vi "JTAG Stim ASIC SPI Test.vi"(5 "Test Type":u16(ring) items=["SPI Self Test", "Stim Register Test", "Stim RAM Test"], 11 "error in (no error)":errorcluster) -> (6 "Test Result":string, 15 "error out":errorcluster)   [LabVIEW 2010]
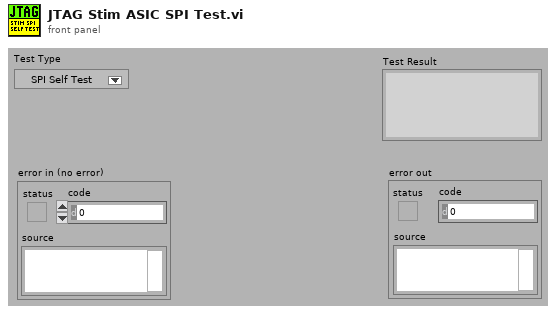
[diagram p1: front panel]
types:
  T1 = enum16{"Read General Control Registers", "Read Phase Registers", "Read RAM1", "Read RAM2", "WE Test0", "WE Test1", "WE Test2", "WE Test3", "WE Test4", "WE Test5", "WE Test6", "WE Test7", "Address Bus Test", "General Register 1's and 0's", "General Register 1's and 0's Inverse", "Phase Register 1's and 0's", "Phase Register 1's and 0's Inverse", "RAM1 data bus 0", "RAM1 data bus 1", "RAM1 data bus 2", "RAM1 data bus 3", "RAM1 data bus 4", "RAM1 data bus 5", "RAM1 data bus 6", "RAM1 data bus 7", "RAM2 data bus 0", "RAM2 data bus 1", "RAM2 data bus 2", "RAM2 data bus 3", "RAM2 data bus 4", "RAM2 data bus 5", "RAM2 data bus 6", "RAM2 data bus 7", "RAM Address Bus Test", "RAM 1's and 0's", "RAM 1's and 0's Inverse", "Address Decoder Test"}[]
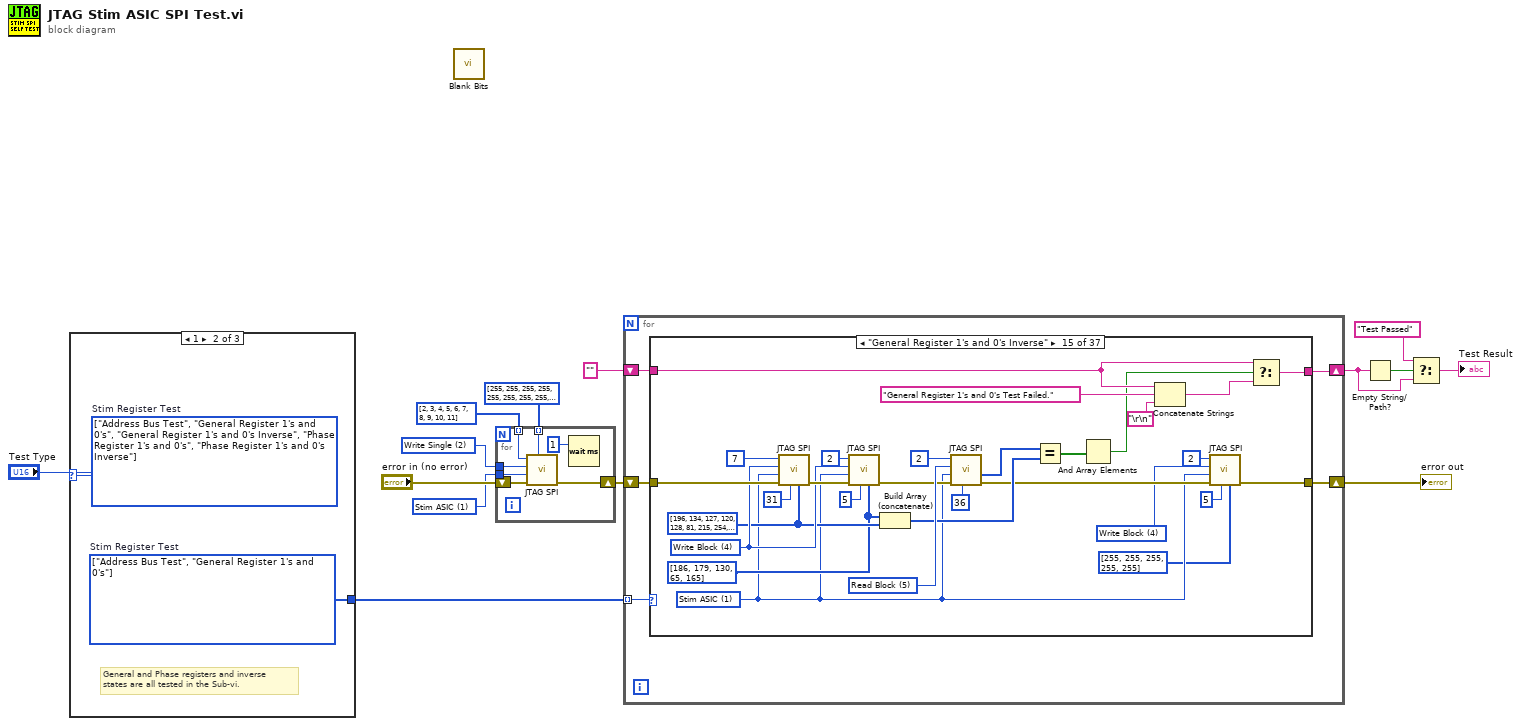
[diagram p0: block diagram]
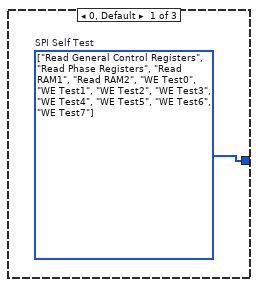
[diagram p2: hidden frame]
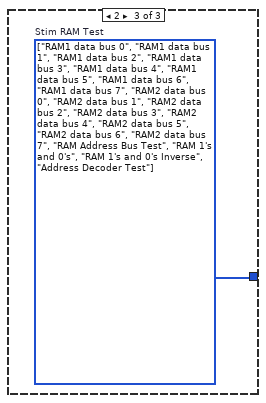
[diagram p3: hidden frame]
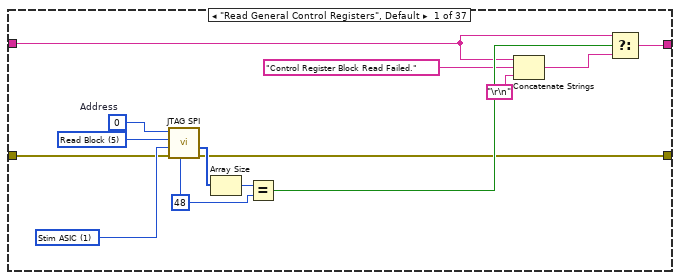
[diagram p4: hidden frame]
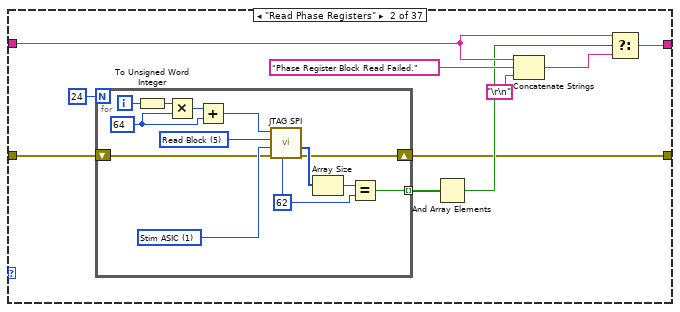
[diagram p5: hidden frame]
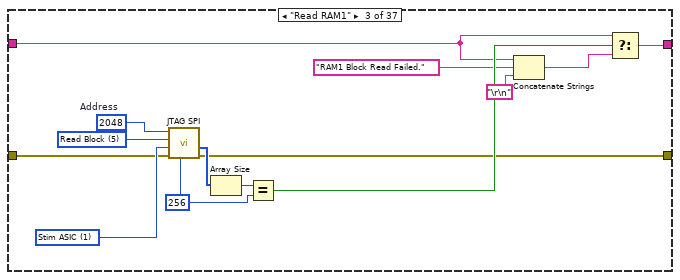
[diagram p6: hidden frame]
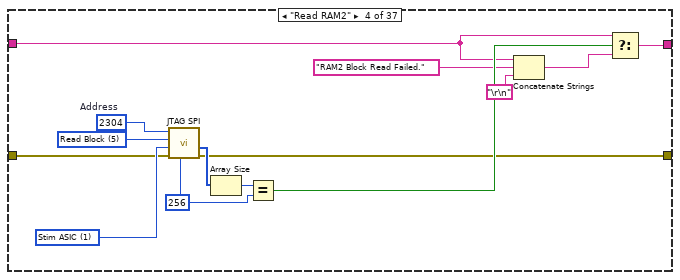
[diagram p7: hidden frame]
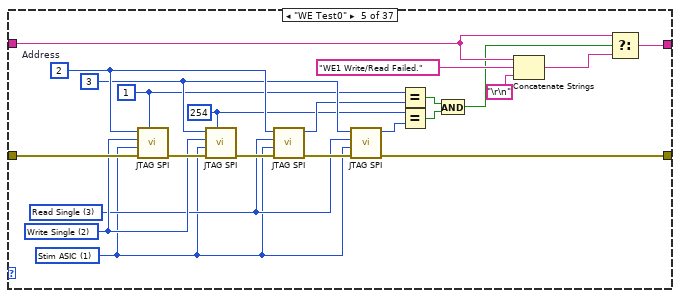
[diagram p8: hidden frame]
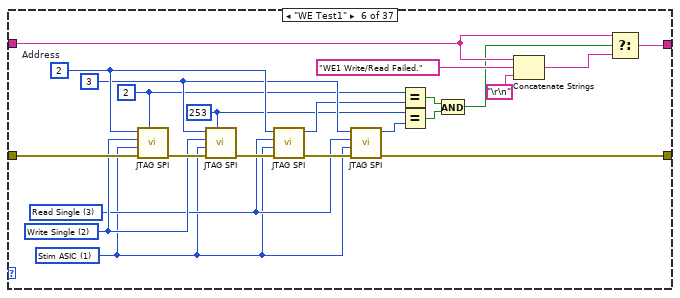
[diagram p9: hidden frame]
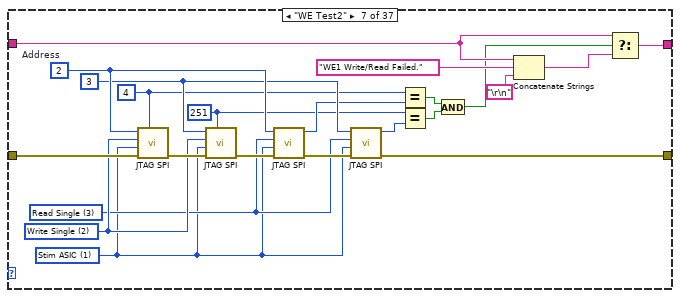
[diagram p10: hidden frame]
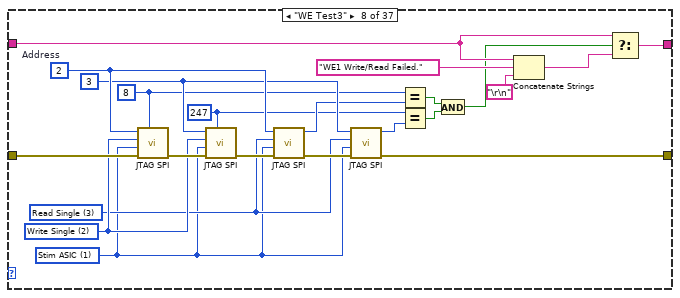
[diagram p11: hidden frame]
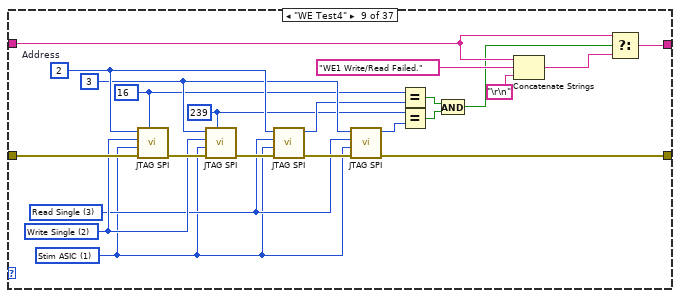
[diagram p12: hidden frame]
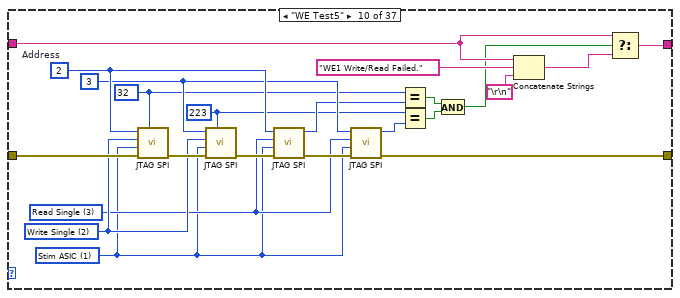
[diagram p13: hidden frame]
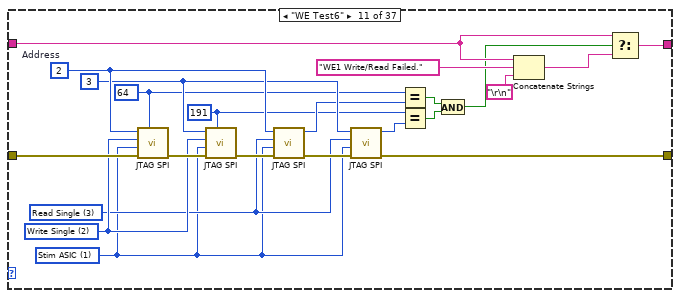
[diagram p14: hidden frame]
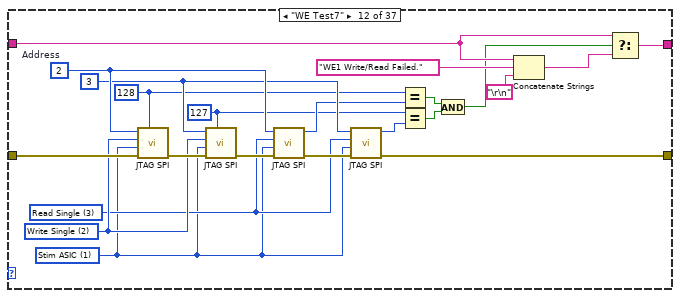
[diagram p15: hidden frame]
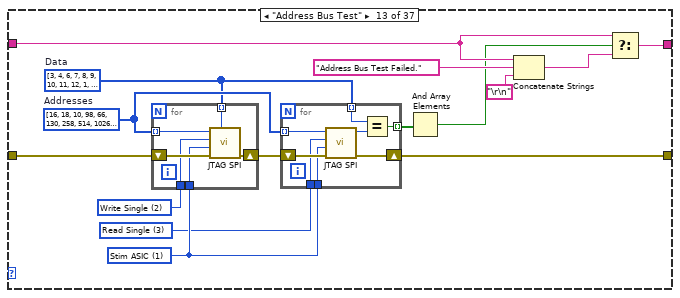
[diagram p16: hidden frame]
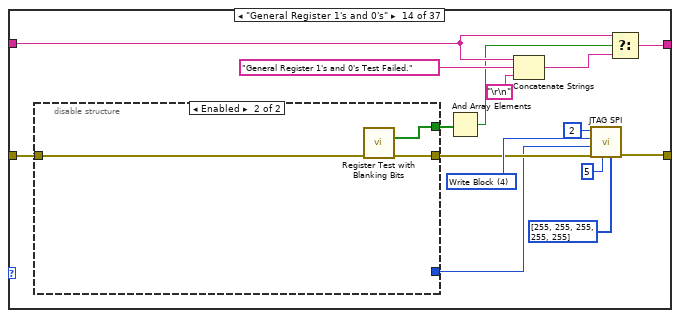
[diagram p17: hidden frame]
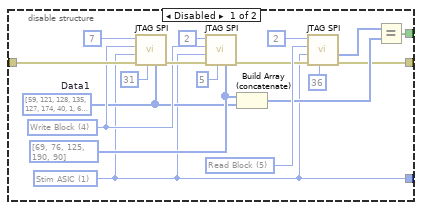
[diagram p18: hidden frame]
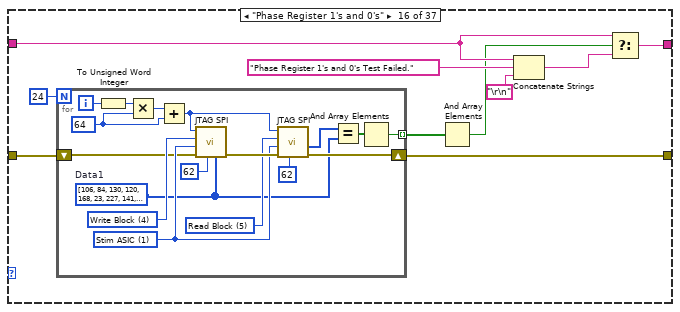
[diagram p19: hidden frame]
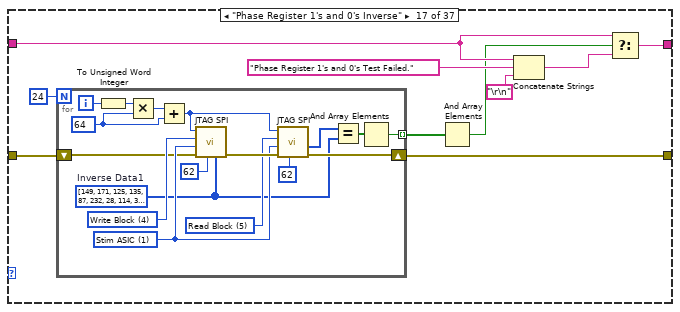
[diagram p20: hidden frame]
diagram:
  w4 = u16 2 items=["Power UP", "Power DN", "Write Single", "Read Single", "Write Block", "Read Block", "Write Masked", "Test Value"] ("Function")
  w5 = u16 1 items=["Power ASIC", "Stim ASIC", "MICS Radio", "FRAM"] ("Target")
  n1 = case shown="1" "Test Type" {
    tunnel: [w15 w16 w17] -> w7
    frame 0, Default {
      w15 = T1 [enum."Read General Control Registers", enum."Read Phase Registers", enum."Read RAM1", enum."Read RAM2", enum."WE Test0", enum."WE Test1", enum."WE Test2", enum."WE Test3", enum."WE Test4", enum."WE Test5", enum."WE Test6", enum."WE Test7"] items=["Read General Control Registers", "Read Phase Registers", "Read RAM1", "Read RAM2", "WE Test0", "WE Test1", "WE Test2", "WE Test3", "WE Test4", "WE Test5", "WE Test6", "WE Test7", "Address Bus Test", "General Register 1's and 0's", "General Register 1's and 0's Inverse", "Phase Register 1's and 0's", "Phase Register 1's and 0's Inverse", "RAM1 data bus 0", "RAM1 data bus 1", "RAM1 data bus 2", "RAM1 data bus 3", "RAM1 data bus 4", "RAM1 data bus 5", "RAM1 data bus 6", "RAM1 data bus 7", "RAM2 data bus 0", "RAM2 data bus 1", "RAM2 data bus 2", "RAM2 data bus 3", "RAM2 data bus 4", "RAM2 data bus 5", "RAM2 data bus 6", "RAM2 data bus 7", "RAM Address Bus Test", "RAM 1's and 0's", "RAM 1's and 0's Inverse", "Address Decoder Test"]  # SPI Self Test
    }
    frame 1 {
      (unwired) T1 [enum."Address Bus Test", enum."General Register 1's and 0's", enum."General Register 1's and 0's Inverse", enum."Phase Register 1's and 0's", enum."Phase Register 1's and 0's Inverse"] items=["Read General Control Registers", "Read Phase Registers", "Read RAM1", "Read RAM2", "WE Test0", "WE Test1", "WE Test2", "WE Test3", "WE Test4", "WE Test5", "WE Test6", "WE Test7", "Address Bus Test", "General Register 1's and 0's", "General Register 1's and 0's Inverse", "Phase Register 1's and 0's", "Phase Register 1's and 0's Inverse", "RAM1 data bus 0", "RAM1 data bus 1", "RAM1 data bus 2", "RAM1 data bus 3", "RAM1 data bus 4", "RAM1 data bus 5", "RAM1 data bus 6", "RAM1 data bus 7", "RAM2 data bus 0", "RAM2 data bus 1", "RAM2 data bus 2", "RAM2 data bus 3", "RAM2 data bus 4", "RAM2 data bus 5", "RAM2 data bus 6", "RAM2 data bus 7", "RAM Address Bus Test", "RAM 1's and 0's", "RAM 1's and 0's Inverse", "Address Decoder Test"]  # Stim Register Test
      w16 = T1 [enum."Address Bus Test", enum."General Register 1's and 0's"] items=["Read General Control Registers", "Read Phase Registers", "Read RAM1", "Read RAM2", "WE Test0", "WE Test1", "WE Test2", "WE Test3", "WE Test4", "WE Test5", "WE Test6", "WE Test7", "Address Bus Test", "General Register 1's and 0's", "General Register 1's and 0's Inverse", "Phase Register 1's and 0's", "Phase Register 1's and 0's Inverse", "RAM1 data bus 0", "RAM1 data bus 1", "RAM1 data bus 2", "RAM1 data bus 3", "RAM1 data bus 4", "RAM1 data bus 5", "RAM1 data bus 6", "RAM1 data bus 7", "RAM2 data bus 0", "RAM2 data bus 1", "RAM2 data bus 2", "RAM2 data bus 3", "RAM2 data bus 4", "RAM2 data bus 5", "RAM2 data bus 6", "RAM2 data bus 7", "RAM Address Bus Test", "RAM 1's and 0's", "RAM 1's and 0's Inverse", "Address Decoder Test"]  # Stim Register Test
      # "General and Phase registers and inverse\nstates are all tested in the Sub-vi."
    }
    frame 2 {
      w17 = T1 [enum."RAM1 data bus 0", enum."RAM1 data bus 1", enum."RAM1 data bus 2", enum."RAM1 data bus 3", enum."RAM1 data bus 4", enum."RAM1 data bus 5", enum."RAM1 data bus 6", enum."RAM1 data bus 7", enum."RAM2 data bus 0", enum."RAM2 data bus 1", enum."RAM2 data bus 2", enum."RAM2 data bus 3", enum."RAM2 data bus 4", enum."RAM2 data bus 5", enum."RAM2 data bus 6", enum."RAM2 data bus 7", enum."RAM Address Bus Test", enum."RAM 1's and 0's", enum."RAM 1's and 0's Inverse", enum."Address Decoder Test"] items=["Read General Control Registers", "Read Phase Registers", "Read RAM1", "Read RAM2", "WE Test0", "WE Test1", "WE Test2", "WE Test3", "WE Test4", "WE Test5", "WE Test6", "WE Test7", "Address Bus Test", "General Register 1's and 0's", "General Register 1's and 0's Inverse", "Phase Register 1's and 0's", "Phase Register 1's and 0's Inverse", "RAM1 data bus 0", "RAM1 data bus 1", "RAM1 data bus 2", "RAM1 data bus 3", "RAM1 data bus 4", "RAM1 data bus 5", "RAM1 data bus 6", "RAM1 data bus 7", "RAM2 data bus 0", "RAM2 data bus 1", "RAM2 data bus 2", "RAM2 data bus 3", "RAM2 data bus 4", "RAM2 data bus 5", "RAM2 data bus 6", "RAM2 data bus 7", "RAM Address Bus Test", "RAM 1's and 0's", "RAM 1's and 0's Inverse", "Address Decoder Test"]  # Stim RAM Test
    }
  }
  n2 = call "Blank Bits.vi"() -> ()  [unwired: 14 in, 2 out]
  n3 = for {
    tunnel: w5 -> [w22]
    tunnel: w4 -> [w21]
    shift-right: [w23] -> w1
    shift-left: "error in (no error)" -> [w24]
    tunnel: u8[] [255, 255, 255, 255, 255, 255, 255, 255, 63, 3] ("Block Write Data") -> [w20] mode=indexing
    tunnel: u16[] [2, 3, 4, 5, 6, 7, 8, 9, 10, 11] ("Block Write Data") -> [w19] mode=indexing
    n4 = call "JTAG SPI.vi"("Value"=w20, "error in (no error)"=w24, "Target"=w22, "Function"=w21, "Address"=w19) -> ("error out"=w23:errorcluster)  [unwired: 3 in, 3 out]
    n5 = Wait (ms)(milliseconds to wait=u32 1) -> ()  [unwired: 1 out]
  }
  n6 = for {
    tunnel: w7 -> [w29] mode=indexing
    shift-right: [w27] -> w11
    shift-left: "" -> [w26]
    shift-right: [w25] -> w13
    shift-left: w1 -> [w28]
    n7 = case shown="\"General Register 1's and 0's Inverse\"" w29 {
      tunnel: w28 -> [w37 w53 w74 w88 w116 w138 w160 w182 w204 w226 w248 w270 w285 w314 w364 w367 w394 w440 w462 w484 w506 w528 w550 w572 w594 w616 w638 w660 w682 w704 w726 w748 w770 w785 w813 w831 w865]
      tunnel: [w30 w44 w67 w81 w106 w128 w150 w172 w194 w216 w238 w260 w275 w301 w339 w366 w393 w430 w452 w474 w496 w518 w540 w562 w584 w606 w628 w650 w672 w694 w716 w738 w760 w775 w812 w830 w852] -> w25
      tunnel: [w36 w52 w73 w87 w115 w137 w159 w181 w203 w225 w247 w269 w284 w313 w363 w374 w401 w439 w461 w483 w505 w527 w549 w571 w593 w615 w637 w659 w681 w703 w725 w747 w769 w784 w819 w837 w864] -> w27
      tunnel: w26 -> [w34 w50 w71 w85 w113 w135 w157 w179 w201 w223 w245 w267 w283 w312 w362 w373 w400 w437 w459 w481 w503 w525 w547 w569 w591 w613 w635 w657 w679 w701 w723 w745 w767 w783 w818 w836 w863]
      frame "Read General Control Registers", Default {
        w38 = u16 48 ("Blocksize")
        w41 = u16 1 items=["Power ASIC", "Stim ASIC", "MICS Radio", "FRAM"] ("Target")
        w42 = u16 5 items=["Power UP", "Power DN", "Write Single", "Read Single", "Write Block", "Read Block", "Write Masked", "Test Value"] ("Function")
        w43 = u16 0  # Address
        n8 = call "JTAG SPI.vi"("Blocksize"=w38, "error in (no error)"=w37, "Target"=w41, "Function"=w42, "Address"=w43) -> ("error out"=w30:errorcluster, "Block Read Data"=w40:u16[])  [unwired: 3 in, 2 out]
        n9 = Array Size(array=w40) -> (size(s)=w39:i32)
        n10 = Equal?(x=w39, y=w38) -> (x = y?=w35:bool)
        n11 = Concatenate Strings(w34, "Control Register Block Read Failed." ("string"), "\r\n") -> (w33:string)
        n12 = Select(t=w34, s=w35, f=w33) -> (s? t:f=w36:string)
      }
      frame "Read Phase Registers" {
        n13 = for {
          N: 24 -> [_]
          tunnel: [w59] -> w51 mode=indexing
          shift-right: [w60] -> w44
          shift-left: w53 -> [w61]
          i -> [w58]
          w55 = u16 64 ("y")
          w62 = u16 62 ("Blocksize")
          w65 = u16 1 items=["Power ASIC", "Stim ASIC", "MICS Radio", "FRAM"] ("Target")
          w66 = u16 5 items=["Power UP", "Power DN", "Write Single", "Read Single", "Write Block", "Read Block", "Write Masked", "Test Value"] ("Function")
          n14 = To Unsigned Word Integer(number=w58) -> (unsigned 16bit integer=w57:u16)
          n15 = Multiply(x=w57, y=w55) -> (x*y=w56:u16)
          n16 = Add(x=w56, y=w55) -> (x+y=w54:u16)
          n17 = call "JTAG SPI.vi"("Blocksize"=w62, "error in (no error)"=w61, "Target"=w65, "Function"=w66, "Address"=w54) -> ("error out"=w60:errorcluster, "Block Read Data"=w64:u16[])  [unwired: 3 in, 2 out]
          n18 = Array Size(array=w64) -> (size(s)=w63:i32)
          n19 = Equal?(x=w63, y=w62) -> (x = y?=w59:bool)
        }
        n20 = And Array Elements(Boolean array=w51) -> (logical AND=w46:bool)
        n21 = Concatenate Strings(w50, "Phase Register Block Read Failed." ("string"), "\r\n") -> (w49:string)
        n22 = Select(t=w50, s=w46, f=w49) -> (s? t:f=w52:string)
      }
      frame "Read RAM1" {
        w75 = u16 256 ("Blocksize")
        w78 = u16 1 items=["Power ASIC", "Stim ASIC", "MICS Radio", "FRAM"] ("Target")
        w79 = u16 5 items=["Power UP", "Power DN", "Write Single", "Read Single", "Write Block", "Read Block", "Write Masked", "Test Value"] ("Function")
        w80 = u16 2048  # Address
        n23 = call "JTAG SPI.vi"("Blocksize"=w75, "error in (no error)"=w74, "Target"=w78, "Function"=w79, "Address"=w80) -> ("error out"=w67:errorcluster, "Block Read Data"=w77:u16[])  [unwired: 3 in, 2 out]
        n24 = Array Size(array=w77) -> (size(s)=w76:i32)
        n25 = Equal?(x=w76, y=w75) -> (x = y?=w72:bool)
        n26 = Concatenate Strings(w71, "RAM1 Block Read Failed." ("string"), "\r\n") -> (w70:string)
        n27 = Select(t=w71, s=w72, f=w70) -> (s? t:f=w73:string)
      }
      frame "Read RAM2" {
        w89 = u16 256 ("Blocksize")
        w92 = u16 1 items=["Power ASIC", "Stim ASIC", "MICS Radio", "FRAM"] ("Target")
        w93 = u16 5 items=["Power UP", "Power DN", "Write Single", "Read Single", "Write Block", "Read Block", "Write Masked", "Test Value"] ("Function")
        w94 = u16 2304  # Address
        n28 = call "JTAG SPI.vi"("Blocksize"=w89, "error in (no error)"=w88, "Target"=w92, "Function"=w93, "Address"=w94) -> ("error out"=w81:errorcluster, "Block Read Data"=w91:u16[])  [unwired: 3 in, 2 out]
        n29 = Array Size(array=w91) -> (size(s)=w90:i32)
        n30 = Equal?(x=w90, y=w89) -> (x = y?=w86:bool)
        n31 = Concatenate Strings(w85, "RAM2 Block Read Failed." ("string"), "\r\n") -> (w84:string)
        n32 = Select(t=w85, s=w86, f=w84) -> (s? t:f=w87:string)
      }
      frame "WE Test0" {
        w98 = u8 254 ("Value")
        w100 = u8 1 ("Value")
        w102 = u16 3 items=["Power UP", "Power DN", "Write Single", "Read Single", "Write Block", "Read Block", "Write Masked", "Test Value"] ("Function")
        w104 = u16 3 ("Address")
        w101 = u16 1 items=["Power ASIC", "Stim ASIC", "MICS Radio", "FRAM"] ("Target")
        w103 = u16 2 items=["Power UP", "Power DN", "Write Single", "Read Single", "Write Block", "Read Block", "Write Masked", "Test Value"] ("Function")
        w105 = u16 2  # Address
        n33 = call "JTAG SPI.vi"("Value"=w100, "error in (no error)"=w116, "Target"=w101, "Function"=w103, "Address"=w105) -> ("error out"=w109:errorcluster)  [unwired: 3 in, 3 out]
        n34 = call "JTAG SPI.vi"("Value"=w98, "error in (no error)"=w109, "Target"=w101, "Function"=w103, "Address"=w104) -> ("error out"=w108:errorcluster)  [unwired: 3 in, 3 out]
        n35 = call "JTAG SPI.vi"("error in (no error)"=w108, "Target"=w101, "Function"=w102, "Address"=w105) -> ("error out"=w107:errorcluster, "Read Value"=w99:u8)  [unwired: 4 in, 2 out]
        n36 = call "JTAG SPI.vi"("error in (no error)"=w107, "Target"=w101, "Function"=w102, "Address"=w104) -> ("error out"=w106:errorcluster, "Read Value"=w97:u8)  [unwired: 4 in, 2 out]
        n37 = Equal?(x=w100, y=w99) -> (x = y?=w95:bool)
        n38 = Equal?(x=w98, y=w97) -> (x = y?=w114:bool)
        n39 = And(x=w95, y=w114) -> (x .and. y?=w96:bool)
        n40 = Concatenate Strings(w113, "WE1 Write/Read Failed." ("string"), "\r\n") -> (w112:string)
        n41 = Select(t=w113, s=w96, f=w112) -> (s? t:f=w115:string)
      }
      frame "WE Test1" {
        w120 = u8 253 ("Value")
        w122 = u8 2 ("Value")
        w124 = u16 3 items=["Power UP", "Power DN", "Write Single", "Read Single", "Write Block", "Read Block", "Write Masked", "Test Value"] ("Function")
        w126 = u16 3 ("Address")
        w123 = u16 1 items=["Power ASIC", "Stim ASIC", "MICS Radio", "FRAM"] ("Target")
        w125 = u16 2 items=["Power UP", "Power DN", "Write Single", "Read Single", "Write Block", "Read Block", "Write Masked", "Test Value"] ("Function")
        w127 = u16 2  # Address
        n42 = call "JTAG SPI.vi"("Value"=w122, "error in (no error)"=w138, "Target"=w123, "Function"=w125, "Address"=w127) -> ("error out"=w131:errorcluster)  [unwired: 3 in, 3 out]
        n43 = call "JTAG SPI.vi"("Value"=w120, "error in (no error)"=w131, "Target"=w123, "Function"=w125, "Address"=w126) -> ("error out"=w130:errorcluster)  [unwired: 3 in, 3 out]
        n44 = call "JTAG SPI.vi"("error in (no error)"=w130, "Target"=w123, "Function"=w124, "Address"=w127) -> ("error out"=w129:errorcluster, "Read Value"=w121:u8)  [unwired: 4 in, 2 out]
        n45 = call "JTAG SPI.vi"("error in (no error)"=w129, "Target"=w123, "Function"=w124, "Address"=w126) -> ("error out"=w128:errorcluster, "Read Value"=w119:u8)  [unwired: 4 in, 2 out]
        n46 = Equal?(x=w122, y=w121) -> (x = y?=w117:bool)
        n47 = Equal?(x=w120, y=w119) -> (x = y?=w136:bool)
        n48 = And(x=w117, y=w136) -> (x .and. y?=w118:bool)
        n49 = Concatenate Strings(w135, "WE1 Write/Read Failed." ("string"), "\r\n") -> (w134:string)
        n50 = Select(t=w135, s=w118, f=w134) -> (s? t:f=w137:string)
      }
      frame "WE Test2" {
        w142 = u8 251 ("Value")
        w144 = u8 4 ("Value")
        w146 = u16 3 items=["Power UP", "Power DN", "Write Single", "Read Single", "Write Block", "Read Block", "Write Masked", "Test Value"] ("Function")
        w148 = u16 3 ("Address")
        w145 = u16 1 items=["Power ASIC", "Stim ASIC", "MICS Radio", "FRAM"] ("Target")
        w147 = u16 2 items=["Power UP", "Power DN", "Write Single", "Read Single", "Write Block", "Read Block", "Write Masked", "Test Value"] ("Function")
        w149 = u16 2  # Address
        n51 = call "JTAG SPI.vi"("Value"=w144, "error in (no error)"=w160, "Target"=w145, "Function"=w147, "Address"=w149) -> ("error out"=w153:errorcluster)  [unwired: 3 in, 3 out]
        n52 = call "JTAG SPI.vi"("Value"=w142, "error in (no error)"=w153, "Target"=w145, "Function"=w147, "Address"=w148) -> ("error out"=w152:errorcluster)  [unwired: 3 in, 3 out]
        n53 = call "JTAG SPI.vi"("error in (no error)"=w152, "Target"=w145, "Function"=w146, "Address"=w149) -> ("error out"=w151:errorcluster, "Read Value"=w143:u8)  [unwired: 4 in, 2 out]
        n54 = call "JTAG SPI.vi"("error in (no error)"=w151, "Target"=w145, "Function"=w146, "Address"=w148) -> ("error out"=w150:errorcluster, "Read Value"=w141:u8)  [unwired: 4 in, 2 out]
        n55 = Equal?(x=w144, y=w143) -> (x = y?=w139:bool)
        n56 = Equal?(x=w142, y=w141) -> (x = y?=w158:bool)
        n57 = And(x=w139, y=w158) -> (x .and. y?=w140:bool)
        n58 = Concatenate Strings(w157, "WE1 Write/Read Failed." ("string"), "\r\n") -> (w156:string)
        n59 = Select(t=w157, s=w140, f=w156) -> (s? t:f=w159:string)
      }
      frame "WE Test3" {
        w164 = u8 247 ("Value")
        w166 = u8 8 ("Value")
        w168 = u16 3 items=["Power UP", "Power DN", "Write Single", "Read Single", "Write Block", "Read Block", "Write Masked", "Test Value"] ("Function")
        w170 = u16 3 ("Address")
        w167 = u16 1 items=["Power ASIC", "Stim ASIC", "MICS Radio", "FRAM"] ("Target")
        w169 = u16 2 items=["Power UP", "Power DN", "Write Single", "Read Single", "Write Block", "Read Block", "Write Masked", "Test Value"] ("Function")
        w171 = u16 2  # Address
        n60 = call "JTAG SPI.vi"("Value"=w166, "error in (no error)"=w182, "Target"=w167, "Function"=w169, "Address"=w171) -> ("error out"=w175:errorcluster)  [unwired: 3 in, 3 out]
        n61 = call "JTAG SPI.vi"("Value"=w164, "error in (no error)"=w175, "Target"=w167, "Function"=w169, "Address"=w170) -> ("error out"=w174:errorcluster)  [unwired: 3 in, 3 out]
        n62 = call "JTAG SPI.vi"("error in (no error)"=w174, "Target"=w167, "Function"=w168, "Address"=w171) -> ("error out"=w173:errorcluster, "Read Value"=w165:u8)  [unwired: 4 in, 2 out]
        n63 = call "JTAG SPI.vi"("error in (no error)"=w173, "Target"=w167, "Function"=w168, "Address"=w170) -> ("error out"=w172:errorcluster, "Read Value"=w163:u8)  [unwired: 4 in, 2 out]
        n64 = Equal?(x=w166, y=w165) -> (x = y?=w161:bool)
        n65 = Equal?(x=w164, y=w163) -> (x = y?=w180:bool)
        n66 = And(x=w161, y=w180) -> (x .and. y?=w162:bool)
        n67 = Concatenate Strings(w179, "WE1 Write/Read Failed." ("string"), "\r\n") -> (w178:string)
        n68 = Select(t=w179, s=w162, f=w178) -> (s? t:f=w181:string)
      }
      frame "WE Test4" {
        w186 = u8 239 ("Value")
        w188 = u8 16 ("Value")
        w190 = u16 3 items=["Power UP", "Power DN", "Write Single", "Read Single", "Write Block", "Read Block", "Write Masked", "Test Value"] ("Function")
        w192 = u16 3 ("Address")
        w189 = u16 1 items=["Power ASIC", "Stim ASIC", "MICS Radio", "FRAM"] ("Target")
        w191 = u16 2 items=["Power UP", "Power DN", "Write Single", "Read Single", "Write Block", "Read Block", "Write Masked", "Test Value"] ("Function")
        w193 = u16 2  # Address
        n69 = call "JTAG SPI.vi"("Value"=w188, "error in (no error)"=w204, "Target"=w189, "Function"=w191, "Address"=w193) -> ("error out"=w197:errorcluster)  [unwired: 3 in, 3 out]
        n70 = call "JTAG SPI.vi"("Value"=w186, "error in (no error)"=w197, "Target"=w189, "Function"=w191, "Address"=w192) -> ("error out"=w196:errorcluster)  [unwired: 3 in, 3 out]
        n71 = call "JTAG SPI.vi"("error in (no error)"=w196, "Target"=w189, "Function"=w190, "Address"=w193) -> ("error out"=w195:errorcluster, "Read Value"=w187:u8)  [unwired: 4 in, 2 out]
        n72 = call "JTAG SPI.vi"("error in (no error)"=w195, "Target"=w189, "Function"=w190, "Address"=w192) -> ("error out"=w194:errorcluster, "Read Value"=w185:u8)  [unwired: 4 in, 2 out]
        n73 = Equal?(x=w188, y=w187) -> (x = y?=w183:bool)
        n74 = Equal?(x=w186, y=w185) -> (x = y?=w202:bool)
        n75 = And(x=w183, y=w202) -> (x .and. y?=w184:bool)
        n76 = Concatenate Strings(w201, "WE1 Write/Read Failed." ("string"), "\r\n") -> (w200:string)
        n77 = Select(t=w201, s=w184, f=w200) -> (s? t:f=w203:string)
      }
      frame "WE Test5" {
        w208 = u8 223 ("Value")
        w210 = u8 32 ("Value")
        w212 = u16 3 items=["Power UP", "Power DN", "Write Single", "Read Single", "Write Block", "Read Block", "Write Masked", "Test Value"] ("Function")
        w214 = u16 3 ("Address")
        w211 = u16 1 items=["Power ASIC", "Stim ASIC", "MICS Radio", "FRAM"] ("Target")
        w213 = u16 2 items=["Power UP", "Power DN", "Write Single", "Read Single", "Write Block", "Read Block", "Write Masked", "Test Value"] ("Function")
        w215 = u16 2  # Address
        n78 = call "JTAG SPI.vi"("Value"=w210, "error in (no error)"=w226, "Target"=w211, "Function"=w213, "Address"=w215) -> ("error out"=w219:errorcluster)  [unwired: 3 in, 3 out]
        n79 = call "JTAG SPI.vi"("Value"=w208, "error in (no error)"=w219, "Target"=w211, "Function"=w213, "Address"=w214) -> ("error out"=w218:errorcluster)  [unwired: 3 in, 3 out]
        n80 = call "JTAG SPI.vi"("error in (no error)"=w218, "Target"=w211, "Function"=w212, "Address"=w215) -> ("error out"=w217:errorcluster, "Read Value"=w209:u8)  [unwired: 4 in, 2 out]
        n81 = call "JTAG SPI.vi"("error in (no error)"=w217, "Target"=w211, "Function"=w212, "Address"=w214) -> ("error out"=w216:errorcluster, "Read Value"=w207:u8)  [unwired: 4 in, 2 out]
        n82 = Equal?(x=w210, y=w209) -> (x = y?=w205:bool)
        n83 = Equal?(x=w208, y=w207) -> (x = y?=w224:bool)
        n84 = And(x=w205, y=w224) -> (x .and. y?=w206:bool)
        n85 = Concatenate Strings(w223, "WE1 Write/Read Failed." ("string"), "\r\n") -> (w222:string)
        n86 = Select(t=w223, s=w206, f=w222) -> (s? t:f=w225:string)
      }
      frame "WE Test6" {
        w230 = u8 191 ("Value")
        w232 = u8 64 ("Value")
        w234 = u16 3 items=["Power UP", "Power DN", "Write Single", "Read Single", "Write Block", "Read Block", "Write Masked", "Test Value"] ("Function")
        w236 = u16 3 ("Address")
        w233 = u16 1 items=["Power ASIC", "Stim ASIC", "MICS Radio", "FRAM"] ("Target")
        w235 = u16 2 items=["Power UP", "Power DN", "Write Single", "Read Single", "Write Block", "Read Block", "Write Masked", "Test Value"] ("Function")
        w237 = u16 2  # Address
        n87 = call "JTAG SPI.vi"("Value"=w232, "error in (no error)"=w248, "Target"=w233, "Function"=w235, "Address"=w237) -> ("error out"=w241:errorcluster)  [unwired: 3 in, 3 out]
        n88 = call "JTAG SPI.vi"("Value"=w230, "error in (no error)"=w241, "Target"=w233, "Function"=w235, "Address"=w236) -> ("error out"=w240:errorcluster)  [unwired: 3 in, 3 out]
        n89 = call "JTAG SPI.vi"("error in (no error)"=w240, "Target"=w233, "Function"=w234, "Address"=w237) -> ("error out"=w239:errorcluster, "Read Value"=w231:u8)  [unwired: 4 in, 2 out]
        n90 = call "JTAG SPI.vi"("error in (no error)"=w239, "Target"=w233, "Function"=w234, "Address"=w236) -> ("error out"=w238:errorcluster, "Read Value"=w229:u8)  [unwired: 4 in, 2 out]
        n91 = Equal?(x=w232, y=w231) -> (x = y?=w227:bool)
        n92 = Equal?(x=w230, y=w229) -> (x = y?=w246:bool)
        n93 = And(x=w227, y=w246) -> (x .and. y?=w228:bool)
        n94 = Concatenate Strings(w245, "WE1 Write/Read Failed." ("string"), "\r\n") -> (w244:string)
        n95 = Select(t=w245, s=w228, f=w244) -> (s? t:f=w247:string)
      }
      frame "WE Test7" {
        w252 = u8 127 ("Value")
        w254 = u8 128 ("Value")
        w256 = u16 3 items=["Power UP", "Power DN", "Write Single", "Read Single", "Write Block", "Read Block", "Write Masked", "Test Value"] ("Function")
        w258 = u16 3 ("Address")
        w255 = u16 1 items=["Power ASIC", "Stim ASIC", "MICS Radio", "FRAM"] ("Target")
        w257 = u16 2 items=["Power UP", "Power DN", "Write Single", "Read Single", "Write Block", "Read Block", "Write Masked", "Test Value"] ("Function")
        w259 = u16 2  # Address
        n96 = call "JTAG SPI.vi"("Value"=w254, "error in (no error)"=w270, "Target"=w255, "Function"=w257, "Address"=w259) -> ("error out"=w263:errorcluster)  [unwired: 3 in, 3 out]
        n97 = call "JTAG SPI.vi"("Value"=w252, "error in (no error)"=w263, "Target"=w255, "Function"=w257, "Address"=w258) -> ("error out"=w262:errorcluster)  [unwired: 3 in, 3 out]
        n98 = call "JTAG SPI.vi"("error in (no error)"=w262, "Target"=w255, "Function"=w256, "Address"=w259) -> ("error out"=w261:errorcluster, "Read Value"=w253:u8)  [unwired: 4 in, 2 out]
        n99 = call "JTAG SPI.vi"("error in (no error)"=w261, "Target"=w255, "Function"=w256, "Address"=w258) -> ("error out"=w260:errorcluster, "Read Value"=w251:u8)  [unwired: 4 in, 2 out]
        n100 = Equal?(x=w254, y=w253) -> (x = y?=w249:bool)
        n101 = Equal?(x=w252, y=w251) -> (x = y?=w268:bool)
        n102 = And(x=w249, y=w268) -> (x .and. y?=w250:bool)
        n103 = Concatenate Strings(w267, "WE1 Write/Read Failed." ("string"), "\r\n") -> (w266:string)
        n104 = Select(t=w267, s=w250, f=w266) -> (s? t:f=w269:string)
      }
      frame "Address Bus Test" {
        w274 = u16[] [16, 18, 10, 98, 66, 130, 258, 514, 1026, 2, 3, 6]  # Addresses
        w273 = u8[] [3, 4, 6, 7, 8, 9, 10, 11, 12, 1, 2, 5]  # Data
        w276 = u16 3 items=["Power UP", "Power DN", "Write Single", "Read Single", "Write Block", "Read Block", "Write Masked", "Test Value"] ("Function")
        w277 = u16 1 items=["Power ASIC", "Stim ASIC", "MICS Radio", "FRAM"] ("Target")
        w278 = u16 2 items=["Power UP", "Power DN", "Write Single", "Read Single", "Write Block", "Read Block", "Write Masked", "Test Value"] ("Function")
        n105 = for {
          tunnel: w274 -> [w297] mode=indexing
          tunnel: w278 -> [w296]
          tunnel: w277 -> [w295]
          tunnel: w273 -> [w294] mode=indexing
          shift-right: [w298] -> w279
          shift-left: w285 -> [w299]
          n106 = call "JTAG SPI.vi"("Value"=w294, "error in (no error)"=w299, "Target"=w295, "Function"=w296, "Address"=w297) -> ("error out"=w298:errorcluster)  [unwired: 3 in, 3 out]
        }
        n107 = for {
          tunnel: w277 -> [w292]
          tunnel: w276 -> [w291]
          shift-right: [w290] -> w275
          shift-left: w279 -> [w293]
          tunnel: w274 -> [w289] mode=indexing
          tunnel: w273 -> [w287] mode=indexing
          tunnel: [w286] -> w272 mode=indexing
          n108 = call "JTAG SPI.vi"("error in (no error)"=w293, "Target"=w292, "Function"=w291, "Address"=w289) -> ("error out"=w290:errorcluster, "Read Value"=w288:u8)  [unwired: 4 in, 2 out]
          n109 = Equal?(x=w287, y=w288) -> (x = y?=w286:bool)
        }
        n110 = And Array Elements(Boolean array=w272) -> (logical AND=w271:bool)
        n111 = Concatenate Strings(w283, "Address Bus Test Failed." ("string"), "\r\n") -> (w282:string)
        n112 = Select(t=w283, s=w271, f=w282) -> (s? t:f=w284:string)
      }
      frame "General Register 1's and 0's" {
        w304 = u16 4 items=["Power UP", "Power DN", "Write Single", "Read Single", "Write Block", "Read Block", "Write Masked", "Test Value"] ("Function")
        n113 = disable-structure shown="Enabled" {
          disable-tunnel: w314 -> [w332 w335]
          disable-tunnel: [w330 w333] -> w308
          disable-tunnel: [w316 w334] -> w302
          disable-tunnel: [w315 _] -> w300
          frame Disabled {
            w320 = u8[] [69, 76, 125, 190, 90] ("Data")
            w319 = u8[] [59, 121, 128, 135, 127, 174, 40, 1, 69, 137, 97, 116, 28, 20, 222, 248, 188, 218, 225, 189, 56, 57, 170, 225, 160, 126, 169, 73, 216, 60, 26]  # Data1
            w331 = u16 5 items=["Power UP", "Power DN", "Write Single", "Read Single", "Write Block", "Read Block", "Write Masked", "Test Value"] ("Function")
            w315 = u16 1 items=["Power ASIC", "Stim ASIC", "MICS Radio", "FRAM"] ("Target")
            w325 = u16 4 items=["Power UP", "Power DN", "Write Single", "Read Single", "Write Block", "Read Block", "Write Masked", "Test Value"] ("Function")
            n114 = call "JTAG SPI.vi"("Block Write Data"=w319, "Blocksize"=u16 31, "error in (no error)"=w332, "Target"=w315, "Function"=w325, "Address"=u16 7) -> ("error out"=w327:errorcluster)  [unwired: 2 in, 3 out]
            n115 = call "JTAG SPI.vi"("Block Write Data"=w320, "Blocksize"=u16 5, "error in (no error)"=w327, "Target"=w315, "Function"=w325, "Address"=u16 2) -> ("error out"=w322:errorcluster)  [unwired: 2 in, 3 out]
            n116 = Build Array (concatenate)(w320, w319) -> (w317:u8[])
            n117 = call "JTAG SPI.vi"("Blocksize"=u16 36, "error in (no error)"=w322, "Target"=w315, "Function"=w331, "Address"=u16 2) -> ("error out"=w316:errorcluster, "Block Read Data"=w318:u16[])  [unwired: 3 in, 2 out]
            n118 = Equal?(x=w318, y=w317) -> (x = y?=w330:bool[])
          }
          frame Enabled {
            n119 = call "Register Test with Blanking Bits.vi"("error in"=w335) -> ("Readback Match?"=w333:bool[], "error out"=w334:errorcluster)  [unwired: 13 in]
          }
        }
        n120 = And Array Elements(Boolean array=w308) -> (logical AND=w307:bool)
        n121 = Concatenate Strings(w312, "General Register 1's and 0's Test Failed." ("string"), "\r\n") -> (w311:string)
        n122 = call "JTAG SPI.vi"("Block Write Data"=u8[] [255, 255, 255, 255, 255] ("Inverse Data2"), "Blocksize"=u16 5, "error in (no error)"=w302, "Target"=w300, "Function"=w304, "Address"=u16 2) -> ("error out"=w301:errorcluster)  [unwired: 2 in, 3 out]
        n123 = Select(t=w312, s=w307, f=w311) -> (s? t:f=w313:string)
      }
      frame "General Register 1's and 0's Inverse" {
        w338 = u16 4 items=["Power UP", "Power DN", "Write Single", "Read Single", "Write Block", "Read Block", "Write Masked", "Test Value"] ("Function")
        w343 = u8[] [186, 179, 130, 65, 165] ("Inverse Data2")
        w344 = u8[] [196, 134, 127, 120, 128, 81, 215, 254, 186, 118, 158, 139, 227, 235, 33, 7, 67, 37, 30, 66, 199, 198, 85, 30, 95, 129, 86, 182, 39, 195, 229] ("Inverse Data1")
        w358 = u16 5 items=["Power UP", "Power DN", "Write Single", "Read Single", "Write Block", "Read Block", "Write Masked", "Test Value"] ("Function")
        w337 = u16 1 items=["Power ASIC", "Stim ASIC", "MICS Radio", "FRAM"] ("Target")
        w351 = u16 4 items=["Power UP", "Power DN", "Write Single", "Read Single", "Write Block", "Read Block", "Write Masked", "Test Value"] ("Function")
        n124 = call "JTAG SPI.vi"("Block Write Data"=w344, "Blocksize"=u16 31, "error in (no error)"=w364, "Target"=w337, "Function"=w351, "Address"=u16 7) -> ("error out"=w353:errorcluster)  [unwired: 2 in, 3 out]
        n125 = call "JTAG SPI.vi"("Block Write Data"=w343, "Blocksize"=u16 5, "error in (no error)"=w353, "Target"=w337, "Function"=w351, "Address"=u16 2) -> ("error out"=w348:errorcluster)  [unwired: 2 in, 3 out]
        n126 = Build Array (concatenate)(w343, w344) -> (w345:u8[])
        n127 = call "JTAG SPI.vi"("Blocksize"=u16 36, "error in (no error)"=w348, "Target"=w337, "Function"=w358, "Address"=u16 2) -> ("error out"=w340:errorcluster, "Block Read Data"=w346:u16[])  [unwired: 3 in, 2 out]
        n128 = Equal?(x=w346, y=w345) -> (x = y?=w357:bool[])
        n129 = And Array Elements(Boolean array=w357) -> (logical AND=w356:bool)
        n130 = Concatenate Strings(w362, "General Register 1's and 0's Test Failed." ("string"), "\r\n") -> (w361:string)
        n131 = call "JTAG SPI.vi"("Block Write Data"=u8[] [255, 255, 255, 255, 255] ("Inverse Data2"), "Blocksize"=u16 5, "error in (no error)"=w340, "Target"=w337, "Function"=w338, "Address"=u16 2) -> ("error out"=w339:errorcluster)  [unwired: 2 in, 3 out]
        n132 = Select(t=w362, s=w356, f=w361) -> (s? t:f=w363:string)
      }
      frame "Phase Register 1's and 0's" {
        n133 = for {
          N: 24 -> [_]
          shift-right: [w379] -> w366
          shift-left: w367 -> [w380]
          tunnel: [w375] -> w365 mode=indexing
          i -> [w391]
          w377 = u8[] [106, 84, 130, 120, 168, 23, 227, 141, 252, 8, 179, 118, 214, 187, 218, 212, 173, 207, 30, 186, 226, 198, 106, 248, 43, 21, 191, 233, 243, 156, 193, 243, 252, 127, 153, 110, 12, 64, 120, 1, 41, 97, 179, 189, 235, 149, 31, 156, 10, 101, 84, 144, 102, 8, 15, 123, 212, 23, 29, 5, 217, 205]  # Data1
          w381 = u16 5 items=["Power UP", "Power DN", "Write Single", "Read Single", "Write Block", "Read Block", "Write Masked", "Test Value"] ("Function")
          w386 = u16 1 items=["Power ASIC", "Stim ASIC", "MICS Radio", "FRAM"] ("Target")
          w383 = u16 4 items=["Power UP", "Power DN", "Write Single", "Read Single", "Write Block", "Read Block", "Write Masked", "Test Value"] ("Function")
          w388 = u16 64 ("y")
          n134 = To Unsigned Word Integer(number=w391) -> (unsigned 16bit integer=w390:u16)
          n135 = Multiply(x=w390, y=w388) -> (x*y=w389:u16)
          n136 = Add(x=w389, y=w388) -> (x+y=w378:u16)
          n137 = call "JTAG SPI.vi"("Block Write Data"=w377, "Blocksize"=u16 62, "error in (no error)"=w380, "Target"=w386, "Function"=w383, "Address"=w378) -> ("error out"=w387:errorcluster)  [unwired: 2 in, 3 out]
          n138 = call "JTAG SPI.vi"("Blocksize"=u16 62, "error in (no error)"=w387, "Target"=w386, "Function"=w381, "Address"=w378) -> ("error out"=w379:errorcluster, "Block Read Data"=w385:u16[])  [unwired: 3 in, 2 out]
          n139 = Equal?(x=w385, y=w377) -> (x = y?=w376:bool[])
          n140 = And Array Elements(Boolean array=w376) -> (logical AND=w375:bool)
        }
        n141 = And Array Elements(Boolean array=w365) -> (logical AND=w369:bool)
        n142 = Concatenate Strings(w373, "Phase Register 1's and 0's Test Failed." ("string"), "\r\n") -> (w372:string)
        n143 = Select(t=w373, s=w369, f=w372) -> (s? t:f=w374:string)
      }
      frame "Phase Register 1's and 0's Inverse" {
        n144 = for {
          N: 24 -> [_]
          shift-right: [w406] -> w393
          shift-left: w394 -> [w407]
          tunnel: [w403] -> w392 mode=indexing
          i -> [w418]
          w402 = u8[] [149, 171, 125, 135, 87, 232, 28, 114, 3, 247, 76, 137, 41, 68, 37, 43, 82, 48, 225, 69, 29, 57, 149, 7, 212, 234, 64, 22, 12, 99, 62, 12, 3, 128, 102, 145, 243, 191, 135, 254, 214, 158, 76, 66, 20, 106, 224, 99, 245, 154, 171, 111, 153, 247, 240, 132, 43, 232, 226, 250, 38, 50]  # Inverse Data1
          w408 = u16 5 items=["Power UP", "Power DN", "Write Single", "Read Single", "Write Block", "Read Block", "Write Masked", "Test Value"] ("Function")
          w413 = u16 1 items=["Power ASIC", "Stim ASIC", "MICS Radio", "FRAM"] ("Target")
          w410 = u16 4 items=["Power UP", "Power DN", "Write Single", "Read Single", "Write Block", "Read Block", "Write Masked", "Test Value"] ("Function")
          w415 = u16 64 ("y")
          n145 = To Unsigned Word Integer(number=w418) -> (unsigned 16bit integer=w417:u16)
          n146 = Multiply(x=w417, y=w415) -> (x*y=w416:u16)
          n147 = Add(x=w416, y=w415) -> (x+y=w405:u16)
          n148 = call "JTAG SPI.vi"("Block Write Data"=w402, "Blocksize"=u16 62, "error in (no error)"=w407, "Target"=w413, "Function"=w410, "Address"=w405) -> ("error out"=w414:errorcluster)  [unwired: 2 in, 3 out]
          n149 = call "JTAG SPI.vi"("Blocksize"=u16 62, "error in (no error)"=w414, "Target"=w413, "Function"=w408, "Address"=w405) -> ("error out"=w406:errorcluster, "Block Read Data"=w412:u16[])  [unwired: 3 in, 2 out]
          n150 = Equal?(x=w412, y=w402) -> (x = y?=w404:bool[])
          n151 = And Array Elements(Boolean array=w404) -> (logical AND=w403:bool)
        }
        n152 = And Array Elements(Boolean array=w392) -> (logical AND=w396:bool)
        n153 = Concatenate Strings(w400, "Phase Register 1's and 0's Test Failed." ("string"), "\r\n") -> (w399:string)
        n154 = Select(t=w400, s=w396, f=w399) -> (s? t:f=w401:string)
      }
      frame "RAM1 data bus 0" {
        w422 = u8 254 ("Value")
        w424 = u8 1 ("Value")
        w426 = u16 3 items=["Power UP", "Power DN", "Write Single", "Read Single", "Write Block", "Read Block", "Write Masked", "Test Value"] ("Function")
        w428 = u16 2049 ("Address")
        w425 = u16 1 items=["Power ASIC", "Stim ASIC", "MICS Radio", "FRAM"] ("Target")
        w427 = u16 2 items=["Power UP", "Power DN", "Write Single", "Read Single", "Write Block", "Read Block", "Write Masked", "Test Value"] ("Function")
        w429 = u16 2048  # Address
        n155 = call "JTAG SPI.vi"("Value"=w424, "error in (no error)"=w440, "Target"=w425, "Function"=w427, "Address"=w429) -> ("error out"=w433:errorcluster)  [unwired: 3 in, 3 out]
        n156 = call "JTAG SPI.vi"("Value"=w422, "error in (no error)"=w433, "Target"=w425, "Function"=w427, "Address"=w428) -> ("error out"=w432:errorcluster)  [unwired: 3 in, 3 out]
        n157 = call "JTAG SPI.vi"("error in (no error)"=w432, "Target"=w425, "Function"=w426, "Address"=w429) -> ("error out"=w431:errorcluster, "Read Value"=w423:u8)  [unwired: 4 in, 2 out]
        n158 = call "JTAG SPI.vi"("error in (no error)"=w431, "Target"=w425, "Function"=w426, "Address"=w428) -> ("error out"=w430:errorcluster, "Read Value"=w421:u8)  [unwired: 4 in, 2 out]
        n159 = Equal?(x=w424, y=w423) -> (x = y?=w419:bool)
        n160 = Equal?(x=w422, y=w421) -> (x = y?=w438:bool)
        n161 = And(x=w419, y=w438) -> (x .and. y?=w420:bool)
        n162 = Concatenate Strings(w437, "RAM1 Data Bus Test Failed." ("string"), "\r\n") -> (w436:string)
        n163 = Select(t=w437, s=w420, f=w436) -> (s? t:f=w439:string)
      }
      frame "RAM1 data bus 1" {
        w444 = u8 253 ("Value")
        w446 = u8 2 ("Value")
        w448 = u16 3 items=["Power UP", "Power DN", "Write Single", "Read Single", "Write Block", "Read Block", "Write Masked", "Test Value"] ("Function")
        w450 = u16 2049 ("Address")
        w447 = u16 1 items=["Power ASIC", "Stim ASIC", "MICS Radio", "FRAM"] ("Target")
        w449 = u16 2 items=["Power UP", "Power DN", "Write Single", "Read Single", "Write Block", "Read Block", "Write Masked", "Test Value"] ("Function")
        w451 = u16 2048  # Address
        n164 = call "JTAG SPI.vi"("Value"=w446, "error in (no error)"=w462, "Target"=w447, "Function"=w449, "Address"=w451) -> ("error out"=w455:errorcluster)  [unwired: 3 in, 3 out]
        n165 = call "JTAG SPI.vi"("Value"=w444, "error in (no error)"=w455, "Target"=w447, "Function"=w449, "Address"=w450) -> ("error out"=w454:errorcluster)  [unwired: 3 in, 3 out]
        n166 = call "JTAG SPI.vi"("error in (no error)"=w454, "Target"=w447, "Function"=w448, "Address"=w451) -> ("error out"=w453:errorcluster, "Read Value"=w445:u8)  [unwired: 4 in, 2 out]
        n167 = call "JTAG SPI.vi"("error in (no error)"=w453, "Target"=w447, "Function"=w448, "Address"=w450) -> ("error out"=w452:errorcluster, "Read Value"=w443:u8)  [unwired: 4 in, 2 out]
        n168 = Equal?(x=w446, y=w445) -> (x = y?=w441:bool)
        n169 = Equal?(x=w444, y=w443) -> (x = y?=w460:bool)
        n170 = And(x=w441, y=w460) -> (x .and. y?=w442:bool)
        n171 = Concatenate Strings(w459, "RAM1 Data Bus Test Failed." ("string"), "\r\n") -> (w458:string)
        n172 = Select(t=w459, s=w442, f=w458) -> (s? t:f=w461:string)
      }
      frame "RAM1 data bus 2" {
        w466 = u8 251 ("Value")
        w468 = u8 4 ("Value")
        w470 = u16 3 items=["Power UP", "Power DN", "Write Single", "Read Single", "Write Block", "Read Block", "Write Masked", "Test Value"] ("Function")
        w472 = u16 2049 ("Address")
        w469 = u16 1 items=["Power ASIC", "Stim ASIC", "MICS Radio", "FRAM"] ("Target")
        w471 = u16 2 items=["Power UP", "Power DN", "Write Single", "Read Single", "Write Block", "Read Block", "Write Masked", "Test Value"] ("Function")
        w473 = u16 2048  # Address
        n173 = call "JTAG SPI.vi"("Value"=w468, "error in (no error)"=w484, "Target"=w469, "Function"=w471, "Address"=w473) -> ("error out"=w477:errorcluster)  [unwired: 3 in, 3 out]
        n174 = call "JTAG SPI.vi"("Value"=w466, "error in (no error)"=w477, "Target"=w469, "Function"=w471, "Address"=w472) -> ("error out"=w476:errorcluster)  [unwired: 3 in, 3 out]
        n175 = call "JTAG SPI.vi"("error in (no error)"=w476, "Target"=w469, "Function"=w470, "Address"=w473) -> ("error out"=w475:errorcluster, "Read Value"=w467:u8)  [unwired: 4 in, 2 out]
        n176 = call "JTAG SPI.vi"("error in (no error)"=w475, "Target"=w469, "Function"=w470, "Address"=w472) -> ("error out"=w474:errorcluster, "Read Value"=w465:u8)  [unwired: 4 in, 2 out]
        n177 = Equal?(x=w468, y=w467) -> (x = y?=w463:bool)
        n178 = Equal?(x=w466, y=w465) -> (x = y?=w482:bool)
        n179 = And(x=w463, y=w482) -> (x .and. y?=w464:bool)
        n180 = Concatenate Strings(w481, "RAM1 Data Bus Test Failed." ("string"), "\r\n") -> (w480:string)
        n181 = Select(t=w481, s=w464, f=w480) -> (s? t:f=w483:string)
      }
      frame "RAM1 data bus 3" {
        w488 = u8 247 ("Value")
        w490 = u8 8 ("Value")
        w492 = u16 3 items=["Power UP", "Power DN", "Write Single", "Read Single", "Write Block", "Read Block", "Write Masked", "Test Value"] ("Function")
        w494 = u16 2049 ("Address")
        w491 = u16 1 items=["Power ASIC", "Stim ASIC", "MICS Radio", "FRAM"] ("Target")
        w493 = u16 2 items=["Power UP", "Power DN", "Write Single", "Read Single", "Write Block", "Read Block", "Write Masked", "Test Value"] ("Function")
        w495 = u16 2048  # Address
        n182 = call "JTAG SPI.vi"("Value"=w490, "error in (no error)"=w506, "Target"=w491, "Function"=w493, "Address"=w495) -> ("error out"=w499:errorcluster)  [unwired: 3 in, 3 out]
        n183 = call "JTAG SPI.vi"("Value"=w488, "error in (no error)"=w499, "Target"=w491, "Function"=w493, "Address"=w494) -> ("error out"=w498:errorcluster)  [unwired: 3 in, 3 out]
        n184 = call "JTAG SPI.vi"("error in (no error)"=w498, "Target"=w491, "Function"=w492, "Address"=w495) -> ("error out"=w497:errorcluster, "Read Value"=w489:u8)  [unwired: 4 in, 2 out]
        n185 = call "JTAG SPI.vi"("error in (no error)"=w497, "Target"=w491, "Function"=w492, "Address"=w494) -> ("error out"=w496:errorcluster, "Read Value"=w487:u8)  [unwired: 4 in, 2 out]
        n186 = Equal?(x=w490, y=w489) -> (x = y?=w485:bool)
        n187 = Equal?(x=w488, y=w487) -> (x = y?=w504:bool)
        n188 = And(x=w485, y=w504) -> (x .and. y?=w486:bool)
        n189 = Concatenate Strings(w503, "RAM1 Data Bus Test Failed." ("string"), "\r\n") -> (w502:string)
        n190 = Select(t=w503, s=w486, f=w502) -> (s? t:f=w505:string)
      }
      frame "RAM1 data bus 4" {
        w510 = u8 239 ("Value")
        w512 = u8 16 ("Value")
        w514 = u16 3 items=["Power UP", "Power DN", "Write Single", "Read Single", "Write Block", "Read Block", "Write Masked", "Test Value"] ("Function")
        w516 = u16 2049 ("Address")
        w513 = u16 1 items=["Power ASIC", "Stim ASIC", "MICS Radio", "FRAM"] ("Target")
        w515 = u16 2 items=["Power UP", "Power DN", "Write Single", "Read Single", "Write Block", "Read Block", "Write Masked", "Test Value"] ("Function")
        w517 = u16 2048  # Address
        n191 = call "JTAG SPI.vi"("Value"=w512, "error in (no error)"=w528, "Target"=w513, "Function"=w515, "Address"=w517) -> ("error out"=w521:errorcluster)  [unwired: 3 in, 3 out]
        n192 = call "JTAG SPI.vi"("Value"=w510, "error in (no error)"=w521, "Target"=w513, "Function"=w515, "Address"=w516) -> ("error out"=w520:errorcluster)  [unwired: 3 in, 3 out]
        n193 = call "JTAG SPI.vi"("error in (no error)"=w520, "Target"=w513, "Function"=w514, "Address"=w517) -> ("error out"=w519:errorcluster, "Read Value"=w511:u8)  [unwired: 4 in, 2 out]
        n194 = call "JTAG SPI.vi"("error in (no error)"=w519, "Target"=w513, "Function"=w514, "Address"=w516) -> ("error out"=w518:errorcluster, "Read Value"=w509:u8)  [unwired: 4 in, 2 out]
        n195 = Equal?(x=w512, y=w511) -> (x = y?=w507:bool)
        n196 = Equal?(x=w510, y=w509) -> (x = y?=w526:bool)
        n197 = And(x=w507, y=w526) -> (x .and. y?=w508:bool)
        n198 = Concatenate Strings(w525, "RAM1 Data Bus Test Failed." ("string"), "\r\n") -> (w524:string)
        n199 = Select(t=w525, s=w508, f=w524) -> (s? t:f=w527:string)
      }
      frame "RAM1 data bus 5" {
        w532 = u8 223 ("Value")
        w534 = u8 32 ("Value")
        w536 = u16 3 items=["Power UP", "Power DN", "Write Single", "Read Single", "Write Block", "Read Block", "Write Masked", "Test Value"] ("Function")
        w538 = u16 2049 ("Address")
        w535 = u16 1 items=["Power ASIC", "Stim ASIC", "MICS Radio", "FRAM"] ("Target")
        w537 = u16 2 items=["Power UP", "Power DN", "Write Single", "Read Single", "Write Block", "Read Block", "Write Masked", "Test Value"] ("Function")
        w539 = u16 2048  # Address
        n200 = call "JTAG SPI.vi"("Value"=w534, "error in (no error)"=w550, "Target"=w535, "Function"=w537, "Address"=w539) -> ("error out"=w543:errorcluster)  [unwired: 3 in, 3 out]
        n201 = call "JTAG SPI.vi"("Value"=w532, "error in (no error)"=w543, "Target"=w535, "Function"=w537, "Address"=w538) -> ("error out"=w542:errorcluster)  [unwired: 3 in, 3 out]
        n202 = call "JTAG SPI.vi"("error in (no error)"=w542, "Target"=w535, "Function"=w536, "Address"=w539) -> ("error out"=w541:errorcluster, "Read Value"=w533:u8)  [unwired: 4 in, 2 out]
        n203 = call "JTAG SPI.vi"("error in (no error)"=w541, "Target"=w535, "Function"=w536, "Address"=w538) -> ("error out"=w540:errorcluster, "Read Value"=w531:u8)  [unwired: 4 in, 2 out]
        n204 = Equal?(x=w534, y=w533) -> (x = y?=w529:bool)
        n205 = Equal?(x=w532, y=w531) -> (x = y?=w548:bool)
        n206 = And(x=w529, y=w548) -> (x .and. y?=w530:bool)
        n207 = Concatenate Strings(w547, "RAM1 Data Bus Test Failed." ("string"), "\r\n") -> (w546:string)
        n208 = Select(t=w547, s=w530, f=w546) -> (s? t:f=w549:string)
      }
      frame "RAM1 data bus 6" {
        w554 = u8 191 ("Value")
        w556 = u8 64 ("Value")
        w558 = u16 3 items=["Power UP", "Power DN", "Write Single", "Read Single", "Write Block", "Read Block", "Write Masked", "Test Value"] ("Function")
        w560 = u16 2049 ("Address")
        w557 = u16 1 items=["Power ASIC", "Stim ASIC", "MICS Radio", "FRAM"] ("Target")
        w559 = u16 2 items=["Power UP", "Power DN", "Write Single", "Read Single", "Write Block", "Read Block", "Write Masked", "Test Value"] ("Function")
        w561 = u16 2048  # Address
        n209 = call "JTAG SPI.vi"("Value"=w556, "error in (no error)"=w572, "Target"=w557, "Function"=w559, "Address"=w561) -> ("error out"=w565:errorcluster)  [unwired: 3 in, 3 out]
        n210 = call "JTAG SPI.vi"("Value"=w554, "error in (no error)"=w565, "Target"=w557, "Function"=w559, "Address"=w560) -> ("error out"=w564:errorcluster)  [unwired: 3 in, 3 out]
        n211 = call "JTAG SPI.vi"("error in (no error)"=w564, "Target"=w557, "Function"=w558, "Address"=w561) -> ("error out"=w563:errorcluster, "Read Value"=w555:u8)  [unwired: 4 in, 2 out]
        n212 = call "JTAG SPI.vi"("error in (no error)"=w563, "Target"=w557, "Function"=w558, "Address"=w560) -> ("error out"=w562:errorcluster, "Read Value"=w553:u8)  [unwired: 4 in, 2 out]
        n213 = Equal?(x=w556, y=w555) -> (x = y?=w551:bool)
        n214 = Equal?(x=w554, y=w553) -> (x = y?=w570:bool)
        n215 = And(x=w551, y=w570) -> (x .and. y?=w552:bool)
        n216 = Concatenate Strings(w569, "RAM1 Data Bus Test Failed." ("string"), "\r\n") -> (w568:string)
        n217 = Select(t=w569, s=w552, f=w568) -> (s? t:f=w571:string)
      }
      frame "RAM1 data bus 7" {
        w576 = u8 127 ("Value")
        w578 = u8 128 ("Value")
        w580 = u16 3 items=["Power UP", "Power DN", "Write Single", "Read Single", "Write Block", "Read Block", "Write Masked", "Test Value"] ("Function")
        w582 = u16 2049 ("Address")
        w579 = u16 1 items=["Power ASIC", "Stim ASIC", "MICS Radio", "FRAM"] ("Target")
        w581 = u16 2 items=["Power UP", "Power DN", "Write Single", "Read Single", "Write Block", "Read Block", "Write Masked", "Test Value"] ("Function")
        w583 = u16 2048  # Address
        n218 = call "JTAG SPI.vi"("Value"=w578, "error in (no error)"=w594, "Target"=w579, "Function"=w581, "Address"=w583) -> ("error out"=w587:errorcluster)  [unwired: 3 in, 3 out]
        n219 = call "JTAG SPI.vi"("Value"=w576, "error in (no error)"=w587, "Target"=w579, "Function"=w581, "Address"=w582) -> ("error out"=w586:errorcluster)  [unwired: 3 in, 3 out]
        n220 = call "JTAG SPI.vi"("error in (no error)"=w586, "Target"=w579, "Function"=w580, "Address"=w583) -> ("error out"=w585:errorcluster, "Read Value"=w577:u8)  [unwired: 4 in, 2 out]
        n221 = call "JTAG SPI.vi"("error in (no error)"=w585, "Target"=w579, "Function"=w580, "Address"=w582) -> ("error out"=w584:errorcluster, "Read Value"=w575:u8)  [unwired: 4 in, 2 out]
        n222 = Equal?(x=w578, y=w577) -> (x = y?=w573:bool)
        n223 = Equal?(x=w576, y=w575) -> (x = y?=w592:bool)
        n224 = And(x=w573, y=w592) -> (x .and. y?=w574:bool)
        n225 = Concatenate Strings(w591, "RAM1 Data Bus Test Failed." ("string"), "\r\n") -> (w590:string)
        n226 = Select(t=w591, s=w574, f=w590) -> (s? t:f=w593:string)
      }
      frame "RAM2 data bus 0" {
        w598 = u8 254 ("Value")
        w600 = u8 1 ("Value")
        w602 = u16 3 items=["Power UP", "Power DN", "Write Single", "Read Single", "Write Block", "Read Block", "Write Masked", "Test Value"] ("Function")
        w604 = u16 2305 ("Address")
        w601 = u16 1 items=["Power ASIC", "Stim ASIC", "MICS Radio", "FRAM"] ("Target")
        w603 = u16 2 items=["Power UP", "Power DN", "Write Single", "Read Single", "Write Block", "Read Block", "Write Masked", "Test Value"] ("Function")
        w605 = u16 2304  # Address
        n227 = call "JTAG SPI.vi"("Value"=w600, "error in (no error)"=w616, "Target"=w601, "Function"=w603, "Address"=w605) -> ("error out"=w609:errorcluster)  [unwired: 3 in, 3 out]
        n228 = call "JTAG SPI.vi"("Value"=w598, "error in (no error)"=w609, "Target"=w601, "Function"=w603, "Address"=w604) -> ("error out"=w608:errorcluster)  [unwired: 3 in, 3 out]
        n229 = call "JTAG SPI.vi"("error in (no error)"=w608, "Target"=w601, "Function"=w602, "Address"=w605) -> ("error out"=w607:errorcluster, "Read Value"=w599:u8)  [unwired: 4 in, 2 out]
        n230 = call "JTAG SPI.vi"("error in (no error)"=w607, "Target"=w601, "Function"=w602, "Address"=w604) -> ("error out"=w606:errorcluster, "Read Value"=w597:u8)  [unwired: 4 in, 2 out]
        n231 = Equal?(x=w600, y=w599) -> (x = y?=w595:bool)
        n232 = Equal?(x=w598, y=w597) -> (x = y?=w614:bool)
        n233 = And(x=w595, y=w614) -> (x .and. y?=w596:bool)
        n234 = Concatenate Strings(w613, "RAM2 Data Bus Test Failed." ("string"), "\r\n") -> (w612:string)
        n235 = Select(t=w613, s=w596, f=w612) -> (s? t:f=w615:string)
      }
      frame "RAM2 data bus 1" {
        w620 = u8 253 ("Value")
        w622 = u8 2 ("Value")
        w624 = u16 3 items=["Power UP", "Power DN", "Write Single", "Read Single", "Write Block", "Read Block", "Write Masked", "Test Value"] ("Function")
        w626 = u16 2305 ("Address")
        w623 = u16 1 items=["Power ASIC", "Stim ASIC", "MICS Radio", "FRAM"] ("Target")
        w625 = u16 2 items=["Power UP", "Power DN", "Write Single", "Read Single", "Write Block", "Read Block", "Write Masked", "Test Value"] ("Function")
        w627 = u16 2304  # Address
        n236 = call "JTAG SPI.vi"("Value"=w622, "error in (no error)"=w638, "Target"=w623, "Function"=w625, "Address"=w627) -> ("error out"=w631:errorcluster)  [unwired: 3 in, 3 out]
        n237 = call "JTAG SPI.vi"("Value"=w620, "error in (no error)"=w631, "Target"=w623, "Function"=w625, "Address"=w626) -> ("error out"=w630:errorcluster)  [unwired: 3 in, 3 out]
        n238 = call "JTAG SPI.vi"("error in (no error)"=w630, "Target"=w623, "Function"=w624, "Address"=w627) -> ("error out"=w629:errorcluster, "Read Value"=w621:u8)  [unwired: 4 in, 2 out]
        n239 = call "JTAG SPI.vi"("error in (no error)"=w629, "Target"=w623, "Function"=w624, "Address"=w626) -> ("error out"=w628:errorcluster, "Read Value"=w619:u8)  [unwired: 4 in, 2 out]
        n240 = Equal?(x=w622, y=w621) -> (x = y?=w617:bool)
        n241 = Equal?(x=w620, y=w619) -> (x = y?=w636:bool)
        n242 = And(x=w617, y=w636) -> (x .and. y?=w618:bool)
        n243 = Concatenate Strings(w635, "RAM2 Data Bus Test Failed." ("string"), "\r\n") -> (w634:string)
        n244 = Select(t=w635, s=w618, f=w634) -> (s? t:f=w637:string)
      }
      frame "RAM2 data bus 2" {
        w642 = u8 251 ("Value")
        w644 = u8 4 ("Value")
        w646 = u16 3 items=["Power UP", "Power DN", "Write Single", "Read Single", "Write Block", "Read Block", "Write Masked", "Test Value"] ("Function")
        w648 = u16 2305 ("Address")
        w645 = u16 1 items=["Power ASIC", "Stim ASIC", "MICS Radio", "FRAM"] ("Target")
        w647 = u16 2 items=["Power UP", "Power DN", "Write Single", "Read Single", "Write Block", "Read Block", "Write Masked", "Test Value"] ("Function")
        w649 = u16 2304  # Address
        n245 = call "JTAG SPI.vi"("Value"=w644, "error in (no error)"=w660, "Target"=w645, "Function"=w647, "Address"=w649) -> ("error out"=w653:errorcluster)  [unwired: 3 in, 3 out]
        n246 = call "JTAG SPI.vi"("Value"=w642, "error in (no error)"=w653, "Target"=w645, "Function"=w647, "Address"=w648) -> ("error out"=w652:errorcluster)  [unwired: 3 in, 3 out]
        n247 = call "JTAG SPI.vi"("error in (no error)"=w652, "Target"=w645, "Function"=w646, "Address"=w649) -> ("error out"=w651:errorcluster, "Read Value"=w643:u8)  [unwired: 4 in, 2 out]
        n248 = call "JTAG SPI.vi"("error in (no error)"=w651, "Target"=w645, "Function"=w646, "Address"=w648) -> ("error out"=w650:errorcluster, "Read Value"=w641:u8)  [unwired: 4 in, 2 out]
        n249 = Equal?(x=w644, y=w643) -> (x = y?=w639:bool)
        n250 = Equal?(x=w642, y=w641) -> (x = y?=w658:bool)
        n251 = And(x=w639, y=w658) -> (x .and. y?=w640:bool)
        n252 = Concatenate Strings(w657, "RAM2 Data Bus Test Failed." ("string"), "\r\n") -> (w656:string)
        n253 = Select(t=w657, s=w640, f=w656) -> (s? t:f=w659:string)
      }
      frame "RAM2 data bus 3" {
        w664 = u8 247 ("Value")
        w666 = u8 8 ("Value")
        w668 = u16 3 items=["Power UP", "Power DN", "Write Single", "Read Single", "Write Block", "Read Block", "Write Masked", "Test Value"] ("Function")
        w670 = u16 2305 ("Address")
        w667 = u16 1 items=["Power ASIC", "Stim ASIC", "MICS Radio", "FRAM"] ("Target")
        w669 = u16 2 items=["Power UP", "Power DN", "Write Single", "Read Single", "Write Block", "Read Block", "Write Masked", "Test Value"] ("Function")
        w671 = u16 2304  # Address
        n254 = call "JTAG SPI.vi"("Value"=w666, "error in (no error)"=w682, "Target"=w667, "Function"=w669, "Address"=w671) -> ("error out"=w675:errorcluster)  [unwired: 3 in, 3 out]
        n255 = call "JTAG SPI.vi"("Value"=w664, "error in (no error)"=w675, "Target"=w667, "Function"=w669, "Address"=w670) -> ("error out"=w674:errorcluster)  [unwired: 3 in, 3 out]
        n256 = call "JTAG SPI.vi"("error in (no error)"=w674, "Target"=w667, "Function"=w668, "Address"=w671) -> ("error out"=w673:errorcluster, "Read Value"=w665:u8)  [unwired: 4 in, 2 out]
        n257 = call "JTAG SPI.vi"("error in (no error)"=w673, "Target"=w667, "Function"=w668, "Address"=w670) -> ("error out"=w672:errorcluster, "Read Value"=w663:u8)  [unwired: 4 in, 2 out]
        n258 = Equal?(x=w666, y=w665) -> (x = y?=w661:bool)
        n259 = Equal?(x=w664, y=w663) -> (x = y?=w680:bool)
        n260 = And(x=w661, y=w680) -> (x .and. y?=w662:bool)
        n261 = Concatenate Strings(w679, "RAM2 Data Bus Test Failed." ("string"), "\r\n") -> (w678:string)
        n262 = Select(t=w679, s=w662, f=w678) -> (s? t:f=w681:string)
      }
      frame "RAM2 data bus 4" {
        w686 = u8 239 ("Value")
        w688 = u8 16 ("Value")
        w690 = u16 3 items=["Power UP", "Power DN", "Write Single", "Read Single", "Write Block", "Read Block", "Write Masked", "Test Value"] ("Function")
        w692 = u16 2305 ("Address")
        w689 = u16 1 items=["Power ASIC", "Stim ASIC", "MICS Radio", "FRAM"] ("Target")
        w691 = u16 2 items=["Power UP", "Power DN", "Write Single", "Read Single", "Write Block", "Read Block", "Write Masked", "Test Value"] ("Function")
        w693 = u16 2304  # Address
        n263 = call "JTAG SPI.vi"("Value"=w688, "error in (no error)"=w704, "Target"=w689, "Function"=w691, "Address"=w693) -> ("error out"=w697:errorcluster)  [unwired: 3 in, 3 out]
        n264 = call "JTAG SPI.vi"("Value"=w686, "error in (no error)"=w697, "Target"=w689, "Function"=w691, "Address"=w692) -> ("error out"=w696:errorcluster)  [unwired: 3 in, 3 out]
        n265 = call "JTAG SPI.vi"("error in (no error)"=w696, "Target"=w689, "Function"=w690, "Address"=w693) -> ("error out"=w695:errorcluster, "Read Value"=w687:u8)  [unwired: 4 in, 2 out]
        n266 = call "JTAG SPI.vi"("error in (no error)"=w695, "Target"=w689, "Function"=w690, "Address"=w692) -> ("error out"=w694:errorcluster, "Read Value"=w685:u8)  [unwired: 4 in, 2 out]
        n267 = Equal?(x=w688, y=w687) -> (x = y?=w683:bool)
        n268 = Equal?(x=w686, y=w685) -> (x = y?=w702:bool)
        n269 = And(x=w683, y=w702) -> (x .and. y?=w684:bool)
        n270 = Concatenate Strings(w701, "RAM2 Data Bus Test Failed." ("string"), "\r\n") -> (w700:string)
        n271 = Select(t=w701, s=w684, f=w700) -> (s? t:f=w703:string)
      }
      frame "RAM2 data bus 5" {
        w708 = u8 223 ("Value")
        w710 = u8 32 ("Value")
        w712 = u16 3 items=["Power UP", "Power DN", "Write Single", "Read Single", "Write Block", "Read Block", "Write Masked", "Test Value"] ("Function")
        w714 = u16 2305 ("Address")
        w711 = u16 1 items=["Power ASIC", "Stim ASIC", "MICS Radio", "FRAM"] ("Target")
        w713 = u16 2 items=["Power UP", "Power DN", "Write Single", "Read Single", "Write Block", "Read Block", "Write Masked", "Test Value"] ("Function")
        w715 = u16 2304  # Address
        n272 = call "JTAG SPI.vi"("Value"=w710, "error in (no error)"=w726, "Target"=w711, "Function"=w713, "Address"=w715) -> ("error out"=w719:errorcluster)  [unwired: 3 in, 3 out]
        n273 = call "JTAG SPI.vi"("Value"=w708, "error in (no error)"=w719, "Target"=w711, "Function"=w713, "Address"=w714) -> ("error out"=w718:errorcluster)  [unwired: 3 in, 3 out]
        n274 = call "JTAG SPI.vi"("error in (no error)"=w718, "Target"=w711, "Function"=w712, "Address"=w715) -> ("error out"=w717:errorcluster, "Read Value"=w709:u8)  [unwired: 4 in, 2 out]
        n275 = call "JTAG SPI.vi"("error in (no error)"=w717, "Target"=w711, "Function"=w712, "Address"=w714) -> ("error out"=w716:errorcluster, "Read Value"=w707:u8)  [unwired: 4 in, 2 out]
        n276 = Equal?(x=w710, y=w709) -> (x = y?=w705:bool)
        n277 = Equal?(x=w708, y=w707) -> (x = y?=w724:bool)
        n278 = And(x=w705, y=w724) -> (x .and. y?=w706:bool)
        n279 = Concatenate Strings(w723, "RAM2 Data Bus Test Failed." ("string"), "\r\n") -> (w722:string)
        n280 = Select(t=w723, s=w706, f=w722) -> (s? t:f=w725:string)
      }
      frame "RAM2 data bus 6" {
        w730 = u8 191 ("Value")
        w732 = u8 64 ("Value")
        w734 = u16 3 items=["Power UP", "Power DN", "Write Single", "Read Single", "Write Block", "Read Block", "Write Masked", "Test Value"] ("Function")
        w736 = u16 2305 ("Address")
        w733 = u16 1 items=["Power ASIC", "Stim ASIC", "MICS Radio", "FRAM"] ("Target")
        w735 = u16 2 items=["Power UP", "Power DN", "Write Single", "Read Single", "Write Block", "Read Block", "Write Masked", "Test Value"] ("Function")
        w737 = u16 2304  # Address
        n281 = call "JTAG SPI.vi"("Value"=w732, "error in (no error)"=w748, "Target"=w733, "Function"=w735, "Address"=w737) -> ("error out"=w741:errorcluster)  [unwired: 3 in, 3 out]
        n282 = call "JTAG SPI.vi"("Value"=w730, "error in (no error)"=w741, "Target"=w733, "Function"=w735, "Address"=w736) -> ("error out"=w740:errorcluster)  [unwired: 3 in, 3 out]
        n283 = call "JTAG SPI.vi"("error in (no error)"=w740, "Target"=w733, "Function"=w734, "Address"=w737) -> ("error out"=w739:errorcluster, "Read Value"=w731:u8)  [unwired: 4 in, 2 out]
        n284 = call "JTAG SPI.vi"("error in (no error)"=w739, "Target"=w733, "Function"=w734, "Address"=w736) -> ("error out"=w738:errorcluster, "Read Value"=w729:u8)  [unwired: 4 in, 2 out]
        n285 = Equal?(x=w732, y=w731) -> (x = y?=w727:bool)
        n286 = Equal?(x=w730, y=w729) -> (x = y?=w746:bool)
        n287 = And(x=w727, y=w746) -> (x .and. y?=w728:bool)
        n288 = Concatenate Strings(w745, "RAM2 Data Bus Test Failed." ("string"), "\r\n") -> (w744:string)
        n289 = Select(t=w745, s=w728, f=w744) -> (s? t:f=w747:string)
      }
      frame "RAM2 data bus 7" {
        w752 = u8 127 ("Value")
        w754 = u8 128 ("Value")
        w756 = u16 3 items=["Power UP", "Power DN", "Write Single", "Read Single", "Write Block", "Read Block", "Write Masked", "Test Value"] ("Function")
        w758 = u16 2305 ("Address")
        w755 = u16 1 items=["Power ASIC", "Stim ASIC", "MICS Radio", "FRAM"] ("Target")
        w757 = u16 2 items=["Power UP", "Power DN", "Write Single", "Read Single", "Write Block", "Read Block", "Write Masked", "Test Value"] ("Function")
        w759 = u16 2304  # Address
        n290 = call "JTAG SPI.vi"("Value"=w754, "error in (no error)"=w770, "Target"=w755, "Function"=w757, "Address"=w759) -> ("error out"=w763:errorcluster)  [unwired: 3 in, 3 out]
        n291 = call "JTAG SPI.vi"("Value"=w752, "error in (no error)"=w763, "Target"=w755, "Function"=w757, "Address"=w758) -> ("error out"=w762:errorcluster)  [unwired: 3 in, 3 out]
        n292 = call "JTAG SPI.vi"("error in (no error)"=w762, "Target"=w755, "Function"=w756, "Address"=w759) -> ("error out"=w761:errorcluster, "Read Value"=w753:u8)  [unwired: 4 in, 2 out]
        n293 = call "JTAG SPI.vi"("error in (no error)"=w761, "Target"=w755, "Function"=w756, "Address"=w758) -> ("error out"=w760:errorcluster, "Read Value"=w751:u8)  [unwired: 4 in, 2 out]
        n294 = Equal?(x=w754, y=w753) -> (x = y?=w749:bool)
        n295 = Equal?(x=w752, y=w751) -> (x = y?=w768:bool)
        n296 = And(x=w749, y=w768) -> (x .and. y?=w750:bool)
        n297 = Concatenate Strings(w767, "RAM2 Data Bus Test Failed." ("string"), "\r\n") -> (w766:string)
        n298 = Select(t=w767, s=w750, f=w766) -> (s? t:f=w769:string)
      }
      frame "RAM Address Bus Test" {
        w772 = u16[] [2048, 2049, 2050, 2052, 2056, 2064, 2080, 2112, 2176, 2304, 2305, 2306, 2308, 2312, 2320, 2336, 2368, 2432]  # Addresses
        w771 = u8[] [1, 2, 3, 4, 5, 6, 7, 8, 9, 255, 254, 253, 252, 251, 250, 249, 248, 247]  # Data
        w776 = u16 3 items=["Power UP", "Power DN", "Write Single", "Read Single", "Write Block", "Read Block", "Write Masked", "Test Value"] ("Function")
        w777 = u16 1 items=["Power ASIC", "Stim ASIC", "MICS Radio", "FRAM"] ("Target")
        w778 = u16 2 items=["Power UP", "Power DN", "Write Single", "Read Single", "Write Block", "Read Block", "Write Masked", "Test Value"] ("Function")
        n299 = for {
          tunnel: w772 -> [w797] mode=indexing
          tunnel: w778 -> [w796]
          tunnel: w777 -> [w795]
          tunnel: w771 -> [w794] mode=indexing
          shift-right: [w798] -> w779
          shift-left: w785 -> [w799]
          n300 = call "JTAG SPI.vi"("Value"=w794, "error in (no error)"=w799, "Target"=w795, "Function"=w796, "Address"=w797) -> ("error out"=w798:errorcluster)  [unwired: 3 in, 3 out]
        }
        n301 = for {
          tunnel: w777 -> [w792]
          tunnel: w776 -> [w791]
          shift-right: [w790] -> w775
          shift-left: w779 -> [w793]
          tunnel: w772 -> [w789] mode=indexing
          tunnel: w771 -> [w787] mode=indexing
          tunnel: [w786] -> w774 mode=indexing
          n302 = call "JTAG SPI.vi"("error in (no error)"=w793, "Target"=w792, "Function"=w791, "Address"=w789) -> ("error out"=w790:errorcluster, "Read Value"=w788:u8)  [unwired: 4 in, 2 out]
          n303 = Equal?(x=w787, y=w788) -> (x = y?=w786:bool)
        }
        n304 = And Array Elements(Boolean array=w774) -> (logical AND=w773:bool)
        n305 = Concatenate Strings(w783, "RAM Address Bus Test Failed." ("string"), "\r\n") -> (w782:string)
        n306 = Select(t=w783, s=w773, f=w782) -> (s? t:f=w784:string)
      }
      frame "RAM 1's and 0's" {
        w802 = u8[] [149, 157, 157, 15, 41, 96, 3, 152, 168, 69, 146, 203, 247, 113, 84, 59, 64, 101, 231, 29, 63, 226, 239, 185, 243, 25, 134, 110, 99, 7, 212, 1, 147, 229, 115, 65, 103, 94, 140, 149, 222, 13, 40, 185, 173, 148, 81, 198, 46, 43, 61, 204, 31, 49, 135, 190, 72, 94, 21, 233, 139, 217, 3, 30, 193, 90, 129, 174, 15, 107, 17, 133, 68, 137, 152, 48, 248, 158, 61, 91, 138, 236, 235, 54, 83, 137, 189, 109, 83, 85, 151, 136, 198, 21, 110, 232, 139, 226, 8, 118, 118, 93, 53, 46, 215, 33, 101, 80, 15, 155, 204, 98, 53, 57, 157, 142, 24, 244, 4, 223, 67, 97, 228, 83, 200, 248, 253, 212, 175, 154, 61, 78, 138, 245, 10, 120, 246, 159, 196, 15, 202, 173, 122, 225, 20, 240, 11, 161, 227, 223, 18, 163, 225, 211, 235, 32, 220, 164, 55, 49, 86, 68, 156, 66, 231, 148, 104, 230, 146, 138, 180, 210, 22, 175, 246, 165, 227, 15, 19, 197, 66, 228, 49, 127, 105, 14, 62, 85, 75, 255, 62, 93, 210, 60, 209, 44, 233, 152, 151, 165, 236, 225, 140, 167, 91, 243, 225, 144, 81, 101, 15, 210, 188, 20, 141, 75, 221, 119, 234, 12, 24, 104, 50, 100, 141, 182, 241, 63, 122, 109, 250, 131, 54, 113, 97, 20, 90, 130, 180, 151, 3, 190, 143, 86, 163, 123, 238, 90, 141, 92, 90, 250, 89, 16, 179, 119, 219, 247, 68, 203, 86, 24, 98, 103, 212, 53, 159, 88, 203, 49, 83, 172, 133, 42, 69, 21, 235, 162, 52, 28, 244, 177, 47, 255, 228, 143, 23, 211, 11, 124, 207, 137, 163, 235, 205, 6, 50, 53, 255, 38, 195, 38, 95, 1, 119, 196, 147, 61, 216, 147, 247, 241, 142, 101, 168, 162, 99, 45, 60, 72, 61, 36, 136, 231, 231, 28, 184, 185, 218, 251, 246, 100, 221, 218, 151, 205, 134, 10, 158, 67, 148, 159, 24, 170, 13, 53, 182, 174, 8, 242, 187, 53, 174, 176, 219, 198, 167, 141, 122, 83, 137, 188, 154, 174, 159, 55, 134, 139, 79, 114, 191, 138, 1, 74, 94, 117, 95, 158, 7, 88, 121, 19, 64, 107, 194, 65, 139, 114, 166, 28, 244, 97, 186, 222, 103, 139, 32, 7, 105, 23, 165, 36, 200, 205, 74, 140, 49, 217, 91, 89, 166, 144, 153, 222, 72, 222, 0, 48, 46, 242, 139, 0, 198, 145, 182, 32, 246, 15, 99, 210, 129, 44, 192, 12, 132, 163, 185, 44, 145, 51, 28, 55, 121, 1, 148, 200, 153, 81, 85, 26, 118, 223, 22, 149, 113, 222, 18, 245, 118, 195, 141, 227, 219, 108, 252, 173, 121, 242, 187, 49, 33, 89, 231, 9, 103, 3, 172, 212, 219, 97, 42, 7, 240, 125, 162, 168, 204, 166, 184, 163, 201, 203, 62, 123, 97, 59, 120, 175, 100, 172, 208, 203, 34, 20, 251, 41, 242, 1, 213, 184, 62, 208]  # Data1
        w805 = u16 5 items=["Power UP", "Power DN", "Write Single", "Read Single", "Write Block", "Read Block", "Write Masked", "Test Value"] ("Function")
        w810 = u16 1 items=["Power ASIC", "Stim ASIC", "MICS Radio", "FRAM"] ("Target")
        w807 = u16 4 items=["Power UP", "Power DN", "Write Single", "Read Single", "Write Block", "Read Block", "Write Masked", "Test Value"] ("Function")
        w804 = u16 2048 ("y")
        n307 = Split 1D Array(array=w802, index=256) -> (first subarray=w801:u8[])  [unwired: 1 out]
        n308 = call "JTAG SPI.vi"("Block Write Data"=w801, "Blocksize"=u16 256, "error in (no error)"=w813, "Target"=w810, "Function"=w807, "Address"=w804) -> ("error out"=w811:errorcluster)  [unwired: 2 in, 3 out]
        n309 = call "JTAG SPI.vi"("Blocksize"=u16 256, "error in (no error)"=w811, "Target"=w810, "Function"=w805, "Address"=w804) -> ("error out"=w812:errorcluster, "Block Read Data"=w809:u16[])  [unwired: 3 in, 2 out]
        n310 = Equal?(x=w809, y=w801) -> (x = y?=w803:bool[])
        n311 = And Array Elements(Boolean array=w803) -> (logical AND=w814:bool)
        n312 = Concatenate Strings(w818, "RAM 1's and 0's Test Failed." ("string"), "\r\n") -> (w817:string)
        n313 = Select(t=w818, s=w814, f=w817) -> (s? t:f=w819:string)
      }
      frame "RAM 1's and 0's Inverse" {
        w820 = u8[] [106, 98, 98, 240, 214, 159, 252, 103, 87, 186, 109, 52, 8, 142, 171, 196, 191, 154, 24, 226, 192, 29, 16, 70, 12, 230, 121, 145, 156, 248, 43, 254, 108, 26, 140, 190, 152, 161, 115, 106, 33, 242, 215, 70, 82, 107, 174, 57, 209, 212, 194, 51, 224, 206, 120, 65, 183, 161, 234, 22, 116, 38, 252, 225, 62, 165, 126, 81, 240, 148, 238, 122, 187, 118, 103, 207, 7, 97, 194, 164, 117, 19, 20, 201, 172, 118, 66, 146, 172, 170, 104, 119, 57, 234, 145, 23, 116, 29, 247, 137, 137, 162, 202, 209, 40, 222, 154, 175, 240, 100, 51, 157, 202, 198, 98, 113, 231, 11, 251, 32, 188, 158, 27, 172, 55, 7, 2, 43, 80, 101, 194, 177, 117, 10, 245, 135, 9, 96, 59, 240, 53, 82, 133, 30, 235, 15, 244, 94, 28, 32, 237, 92, 30, 44, 20, 223, 35, 91, 200, 206, 169, 187, 99, 189, 24, 107, 151, 25, 109, 117, 75, 45, 233, 80, 9, 90, 28, 240, 236, 58, 189, 27, 206, 128, 150, 241, 193, 170, 180, 0, 193, 162, 45, 195, 46, 211, 22, 103, 104, 90, 19, 30, 115, 88, 164, 12, 30, 111, 174, 154, 240, 45, 67, 235, 114, 180, 34, 136, 21, 243, 231, 151, 205, 155, 114, 73, 14, 192, 133, 146, 5, 124, 201, 142, 158, 235, 165, 125, 75, 104, 252, 65, 112, 169, 92, 132, 17, 165, 114, 163, 165, 5, 166, 239, 76, 136, 36, 8, 187, 52, 169, 231, 157, 152, 43, 202, 96, 167, 52, 206, 172, 83, 122, 213, 186, 234, 20, 93, 203, 227, 11, 78, 208, 0, 27, 112, 232, 44, 244, 131, 48, 118, 92, 20, 50, 249, 205, 202, 0, 217, 60, 217, 160, 254, 136, 59, 108, 194, 39, 108, 8, 14, 113, 154, 87, 93, 156, 210, 195, 183, 194, 219, 119, 24, 24, 227, 71, 70, 37, 4, 9, 155, 34, 37, 104, 50, 121, 245, 97, 188, 107, 96, 231, 85, 242, 202, 73, 81, 247, 13, 68, 202, 81, 79, 36, 57, 88, 114, 133, 172, 118, 67, 101, 81, 96, 200, 121, 116, 176, 141, 64, 117, 254, 181, 161, 138, 160, 97, 248, 167, 134, 236, 191, 148, 61, 190, 116, 141, 89, 227, 11, 158, 69, 33, 152, 116, 223, 248, 150, 232, 90, 219, 55, 50, 181, 115, 206, 38, 164, 166, 89, 111, 102, 33, 183, 33, 255, 207, 209, 13, 116, 255, 57, 110, 73, 223, 9, 240, 156, 45, 126, 211, 63, 243, 123, 92, 70, 211, 110, 204, 227, 200, 134, 254, 107, 55, 102, 174, 170, 229, 137, 32, 233, 106, 142, 33, 237, 10, 137, 60, 114, 28, 36, 147, 3, 82, 134, 13, 68, 206, 222, 166, 24, 246, 152, 252, 83, 43, 36, 158, 213, 248, 15, 130, 93, 87, 51, 89, 71, 92, 54, 52, 193, 132, 158, 196, 135, 80, 155, 83, 47, 52, 221, 235, 4, 214, 13, 254, 42, 71, 193, 47]  # Inverse Data1
        w823 = u16 5 items=["Power UP", "Power DN", "Write Single", "Read Single", "Write Block", "Read Block", "Write Masked", "Test Value"] ("Function")
        w828 = u16 1 items=["Power ASIC", "Stim ASIC", "MICS Radio", "FRAM"] ("Target")
        w825 = u16 4 items=["Power UP", "Power DN", "Write Single", "Read Single", "Write Block", "Read Block", "Write Masked", "Test Value"] ("Function")
        w822 = u16 2048 ("y")
        n314 = call "JTAG SPI.vi"("Block Write Data"=w820, "Blocksize"=u16 512, "error in (no error)"=w831, "Target"=w828, "Function"=w825, "Address"=w822) -> ("error out"=w829:errorcluster)  [unwired: 2 in, 3 out]
        n315 = call "JTAG SPI.vi"("Blocksize"=u16 512, "error in (no error)"=w829, "Target"=w828, "Function"=w823, "Address"=w822) -> ("error out"=w830:errorcluster, "Block Read Data"=w827:u16[])  [unwired: 3 in, 2 out]
        n316 = Equal?(x=w827, y=w820) -> (x = y?=w821:bool[])
        n317 = And Array Elements(Boolean array=w821) -> (logical AND=w832:bool)
        n318 = Concatenate Strings(w836, "RAM 1's and 0's Test Failed." ("string"), "\r\n") -> (w835:string)
        n319 = Select(t=w836, s=w832, f=w835) -> (s? t:f=w837:string)
      }
      frame "Address Decoder Test" {
        w845 = u8 19 ("Value")
        w846 = u16 2306 ("Address")
        w855 = u8 18 ("Value")
        w856 = u8 17 ("Value")
        w849 = u16 3 items=["Power UP", "Power DN", "Write Single", "Read Single", "Write Block", "Read Block", "Write Masked", "Test Value"] ("Function")
        w847 = u16 2050 ("Address")
        w851 = u16 1 items=["Power ASIC", "Stim ASIC", "MICS Radio", "FRAM"] ("Target")
        w850 = u16 2 items=["Power UP", "Power DN", "Write Single", "Read Single", "Write Block", "Read Block", "Write Masked", "Test Value"] ("Function")
        w848 = u16 2  # Address
        n320 = call "JTAG SPI.vi"("Value"=w856, "error in (no error)"=w865, "Target"=w851, "Function"=w850, "Address"=w848) -> ("error out"=w859:errorcluster)  [unwired: 3 in, 3 out]
        n321 = call "JTAG SPI.vi"("Value"=w855, "error in (no error)"=w859, "Target"=w851, "Function"=w850, "Address"=w847) -> ("error out"=w858:errorcluster)  [unwired: 3 in, 3 out]
        n322 = call "JTAG SPI.vi"("Value"=w845, "error in (no error)"=w858, "Target"=w851, "Function"=w850, "Address"=w846) -> ("error out"=w857:errorcluster)  [unwired: 3 in, 3 out]
        n323 = call "JTAG SPI.vi"("error in (no error)"=w857, "Target"=w851, "Function"=w849, "Address"=w848) -> ("error out"=w853:errorcluster, "Read Value"=w839:u8)  [unwired: 4 in, 2 out]
        n324 = call "JTAG SPI.vi"("error in (no error)"=w853, "Target"=w851, "Function"=w849, "Address"=w847) -> ("error out"=w854:errorcluster, "Read Value"=w838:u8)  [unwired: 4 in, 2 out]
        n325 = call "JTAG SPI.vi"("error in (no error)"=w854, "Target"=w851, "Function"=w849, "Address"=w846) -> ("error out"=w852:errorcluster, "Read Value"=w844:u8)  [unwired: 4 in, 2 out]
        n326 = Equal?(x=w856, y=w839) -> (x = y?=w842:bool)
        n327 = Equal?(x=w855, y=w838) -> (x = y?=w843:bool)
        n328 = Equal?(x=w845, y=w844) -> (x = y?=w841:bool)
        n329 = Compound Arithmetic op=AND(w842, w843, w841) -> (w840:bool)
        n330 = Concatenate Strings(w863, "Address Decoder Test Failed." ("string"), "\r\n") -> (w862:string)
        n331 = Select(t=w863, s=w840, f=w862) -> (s? t:f=w864:string)
      }
    }
  }
  "error out" <- w13
  n332 = Empty String/Path?(string/path=w11) -> (empty?=w12:bool)
  n333 = Select(t="Test Passed", s=w12, f=w11) -> (s? t:f=→"Test Result":string)
